vi "02 HEWH 24 Hour Test SM1.vi"(0 "Equipment":T1={"COM Port"="COM3", "MW100"="MW100", "AG34970"="A-34972A", "Chamber"="WT500"}, 2 "Semiphore":T2, 11 "Error In":errorcluster) -> (15 "Error Out":errorcluster)   [LabVIEW 2012]
uses:
  EquipReferences.ctl
  HEWH Tank Indicator.ctl
  PowerElements.ctl
  <vilib>/Platform/fileVersionInfo.llb/FileVersionInformation.ctl
  GEA2/HEWH_Mode.ctl
  ChannelSettings.ctl
  ValveBankPositions.ctl
  Intellifaucet/Intellfaucet Mode.ctl
  TestedFlowratesScenarios.ctl
  HEWH Error Enumeration.ctl
  <vilib>/Utility/file.llb/Write To Spreadsheet File (string).vi
  Global HEWH.vi
  <vilib>/Analysis/baseanly.llb/Mean (DBL).vi
  <vilib>/Analysis/NI_AALBase.lvlib
panel:
  in  "Tab Control":enum32{"Page 1", "Page 2"}(tab)
  in  "Time Reset":bool
  in  "Time Update":dbl format="%<%H:%M:%S>t"
  out "Tc Tree Check":dbl[](array[numeric]) format="%.4f"
  out "Serial Data In":string
  in  "IP Agilent":string="192.168.25.2"
  in  "IP MW100":string="192.168.25.4"
  in  "P2":i32=9
  in  "T5 2":i32=9
  in  "T2 2":i32=11
  in  "T1 2":i32=10
  in  "P5":i32=18
  in  "P1":i32=19
  out "Label Array":string[](array[string])
  out "Chanel List":string
  out "Computer Name":string
  in  "Stop Logging":bool
  in  "stop":bool
  out "StopSerial":bool
  out "FileVersionInfo Out":T3
  out "Calibration File Array":dbl[][](array[numeric])
  out "Flow Rate (GPM)":dbl
  out "Degrees F":dbl
  out "Voltage":dbl=240.0
  out "Number of Records":i32
  in  "Stop Test Seqence":bool
  out "Ver.":string
  out "Log Data":string[][](array[string])
  out "DrawCount":i32
  out "POWER":T4
  out "t*=0":dbl format="%<%H:%M:%S>t"
  out "Elapsed.Time (H:M:S)":dbl format="%<%H:%M:%S>t"
  out "STATUS":string
  in  "Help":bool
  out "Tank Display":T5 {"TC6" format="%.2g"; "TIN" format="%.2g"; "TOUT" format="%.2g"; "Mean" format="%.2f"; "Std Dev" format="%.2f"; "TC5" format="%.2g"; "TC4" format="%.2g"; "TC3" format="%.2g"; "TC2" format="%.2g"; "TC1" format="%.2g"}
  out "Current Draw Start Time":dbl format="%.2f"
  out "First Time":bool=TRUE
  out "Current State":string
  out "MW100":refnum<visa-resource-name>
  in  "Tab Control 2":enum32{"TEST STATUS", "DATA VIEW", "R134A P-H"}(tab)
  in  "Status Tabl":T6(tab)=enum."External Program Controls"
  in  "Read Config File":bool
  in  "RTDin to Downspout Offset":dbl
  in  "Power Off Time":dbl=82800.0 format="%<%H:%M>t"
  in  "End Log Duration":dbl=3600.0 format="%<%H:%M>t"
  in  "Config Filename":string="HEWH First Hour Rating.ini"
  in  "Num of PreDraws(0-3)":i32=1
  out "GEA2 HyperData":bool
  out "Data Array":string[][](array[string])
  in  "Expansion Tank?":bool
  out "Dispense Times":dbl[](array[numeric])=[0.0, 3600.0, 7200.0, 10800.0, 14400.0, 18000.0] format="%<%H:%M>t"
  out "Dispense Schedule":dbl[](array[numeric])=[10.72, 10.72, 10.72, 10.72, 10.72, 10.72] format="%.2f"
  out "Flow Rate Schedule":dbl[](array[numeric])=[3.0, 3.0, 3.0, 3.0, 3.0, 3.0] format="%.2f"
  out "Temperature Schedule":dbl[](array[numeric])=[58.0, 58.0, 58.0, 58.0, 58.0, 58.0] format="%.2f"
  in  "Cold Water Available?":bool=TRUE
  in  "T3":u32=500
  in  "T2":u32=150
  out "Local?":bool
  out "LAN IP Address":string="192.168.25.3"
  out "Init Complete":bool=TRUE
  in  "T1":u32=1000
  in  "T4":u32=30
  in  "T5":u32=50
  in  "Purge Guard Time(s)":dbl=360.0
  out "PowerON":bool=TRUE
  in  "Sample Per.(s)":dbl=5.0
  in  "Power Off Guard Time20s)":u32=20
  in  "Working File Directory":path=path "c:/work"
  out "Serial Port Available?":bool=TRUE
  out "COM Port":refnum<visa-resource-name>="COM3"
  in  "Save File Directory":path=path "c:/data"
  out "FileName":path
  out "Use Agilent?":bool
  out "GEA2 Set Mode":T7=enum."HighDemand"
  out "Set PointOut":u8=140
  in  "Calibration File":path=path "C:/work/CalibrationFile.csv"
  out "Calibration File?":bool
  out "Monitoring Temps Chart":T8(graph)
  out "Tcs 1-6":dbl[](array[numeric])
  in  "Purge Right Now":bool
  out "Downspount Flow":dbl(graph)
  out "Downspout Flow":dbl=3.8899999999999997
  out "Downspout Temp":dbl=76.8
  out "Temp Band(+/- F)":dbl=50.0
  out "Flow rate Adj":dbl=85.11482133995038
  out "Downspount Temp":dbl(graph)
  out "TempAdj":dbl
  out "Failed to Start Count":dbl
  in  "RTD Band":dbl=2.0
  in  "Skip Waiting for Cutout":bool
  in  "mean tank upper lim":dbl=140.0
  in  "meant tank lower lim":dbl=130.0
  out "Temp Range Err":bool=TRUE
  out "mean":dbl format="%0.2f"
  in  "Power Off Check Limit":dbl=20.0
  out "M*-1":dbl
  in  "Skip Waiting for Temp 3":bool
  out "Tcs 1-6, Ave. 3":dbl[](array[numeric])
  out "Temps Chart 2":T9(graph)
  in  "Temp Decline Hystersis":dbl=0.2
  out "T_Ave_Max":dbl
  out "T_Ave":dbl
  out "LastDraw":bool=TRUE
  out "T*Max":dbl
  out "Special Last Draw":bool
  out "Discard Last Draw":bool
  out "T*Ave":dbl
  out "T*min":dbl
  out "Volume(Gal.)":dbl
  in  "Flow Adj":dbl=3.0
  in  "Adj Time":dbl=3.0
  in  "K(0.1)":dbl=0.1
  out "TcDown":dbl
  out "Gal Target":dbl
  out "Drawing":bool=TRUE
  out "RTD Out":cluster{dbl, dbl}[](graph)
  out "Flowmeter":cluster{dbl, dbl}[](graph)
  in  "Skip Draw0":bool
  out "TcDown 0":dbl
  out "FlowMeter During Draw0":cluster{dbl, dbl}[](graph)
  out "RTD Out 0":cluster{dbl, dbl}[](graph)
  out "WattHours":dbl
  out "Total Gallons Drawn":dbl
  out "Error History":string[](array[string])
  out "Com History":string[](array[string])
  out "Test Data":dbl[][](array[numeric])
  out "Executaion Sequence":string[](array[string])
  out "Error Datalogging":errorcluster={"status"=TRUE, "code"=-1073807346, "source"="VISA Read in Gather Test Data.vi"}
  out "Serial Error Out":errorcluster
  out "Gallons Chart":dbl(graph)
  out "Temps":T8(graph) caption="Waveform Chart"
  out "Watt Chart":T10(graph)
  out "XY Graph":cluster{dbl[], dbl[]}[](graph)=[{array[3000 elements], array[3000 elements]}, {array[3000 elements], array[3000 elements]}, {array[3000 elements], array[3000 elements]}, {array[3000 elements], array[3000 elements]}, {array[3000 elements], array[3000 elements]}, {array[3000 elements], array[3000 elements]}, {array[3000 elements], array[3000 elements]}, {array[3000 elements], array[3000 elements]}, {array[3000 elements], array[3000 elements]}, {[-20.0, -19.0, -18.0, -17.0, -16.0, -15.0, -14.0, -13.0, -12.0, -11.0, -10.0, -9.0, -8.0, -7.0, -6.0, -5.0, -4.0, -3.0, -2.0, -1.0, 0.0, 1.0, 2.0, 3.0, 4.0, 5.0, 6.0, 7.0, 8.0, 9.0, 10.0, 11.0, 12.0, 13.0, 14.0, 15.0, 16.0, 17.0, 18.0, 19.0, 20.0, 21.0, 22.0, 23.0, 24.0, 25.0, 26.0, 27.0, 28.0, 29.0, 30.0, 31.0, 32.0, 33.0, 34.0, 35.0, 36.0, 37.0, 38.0, 39.0, 40.0, 41.0, 42.0, 43.0, 44.0, 45.0, 46.0, 47.0, 48.0, 49.0, 50.0, 51.0, 52.0, 53.0, 54.0, 55.0, 56.0, 57.0, 58.0, 59.0, 60.0, 61.0, 62.0, 63.0, 64.0, 65.0, 66.0, 67.0, 68.0, 69.0, 70.0, 71.0, 72.0, 73.0, 74.0, 75.0, 76.0, 77.0, 78.0, 79.0, 80.0, 81.0, 82.0, 83.0, 84.0, 85.0, 86.0, 87.0, 88.0, 89.0, 90.0, 91.0, 92.0, 93.0, 94.0, 95.0, 96.0, 97.0, 98.0, 99.0, 100.0, 101.0, 102.0, 103.0, 105.0, 106.0, 107.0, 108.0, 109.0, 110.0, 111.0, 112.0, 113.0, 114.0, 115.0, 116.0, 117.0, 118.0, 119.0, 120.0, 120.0, 119.0, 118.0, 117.0, 116.0, 115.0, 114.0, 113.0, 112.0, 111.0, 110.0, 109.0, 108.0, 107.0, 106.0, 105.0, 104.0, 103.0, 102.0, 101.0, 100.0, 99.0, 98.0, 97.0, 96.0, 95.0, 94.0, 93.0, 92.0, 91.0, 90.0, 89.0, 88.0, 87.0, 86.0, 85.0, 84.0, 83.0, 82.0, 81.0], [0.6289673515895778, 0.7335805994405737, 0.8522944773712947, 0.9865263135707176, 1.1377792235501054, 1.307642283538553, 1.497790359049673, 1.7099835899691802, 1.9460665393720367, 2.2079670150661914, 2.497694574185926, 2.8173387228323223, 3.1690668252624037, 3.5551217379777147, 3.9778191836295544, 4.439544882943048, 4.942751461266441, 5.489955147854285, 6.083732285515876, 6.726715668875549, 7.421590728326429, 8.171091577641509, 8.97799694218748, 9.845125983296143, 10.775334035813131, 11.771508272724029, 12.836563312210393, 13.97343677968726, 15.185084837974983, 16.47447769736936, 17.844595116102667, 19.298421901263723, 20.838943419302854, 22.469141123767677, 24.191988107816766, 26.010444687249684, 27.927454019633004, 29.94593776380572, 32.06879178324577, 34.29888189579838, 36.63903967202567, 39.09205828262364, 41.66068839552788, 44.34763412198737, 47.15554901030907, 50.08703208533592, 53.14462393080051, 56.330802811291676, 59.64798082967107, 63.09850011495871, 66.68462903565818, 70.40855843220261, 74.2723978613939, 78.27817184611749, 82.42781612136012, 86.72317386799375, 91.16599192444974, 95.75791696541866, 100.50049163628815, 105.3951506301971, 110.44321669390614, 115.64589654721868, 121.0042766986882, 126.51931913887094, 132.19185689016396, 138.02258938921167, 144.01207767566953, 150.16073935666577, 156.46884331294888, 162.93650410698515, 169.56367604908513, 176.35014686787835, 183.29553092825122, 190.39926192676901, 197.6605849865805, 205.07854806162732, 212.65199254633424, 220.3795429722877, 228.25959565629924, 236.29030614521017, 244.46957531341766, 252.79503371769874, 261.2640244979903, 269.8735838544667, 278.62041937927586, 287.50088568601166, 296.5109570183827, 305.64619643247437, 314.90172109495234, 324.2721631777093, 333.7516257565242, 343.33363303246585, 353.0110740850571, 362.776139234305, 372.62024791580313, 382.5339667649702, 392.5069163380596, 402.5276645496996, 412.5836045051322, 422.6608138540118, 432.74389199150977, 442.8157709281602, 452.85749412592986, 462.84795675360215, 472.76359917961935, 482.5780439241847, 492.26166554201416, 501.7810808394691, 511.09854992710956, 520.1712821280202, 528.9506547605449, 537.3813812499737, 545.4007215624794, 552.9379365977184, 559.914378684324, 566.2449292917087, 571.841952583963, 576.6234598723152, 580.5270985712426, 583.5301287032851, 585.6703799185226, 587.0558684337939, 587.8482742464494, 588.2187766112756, 588.141222950092, 587.7353480793577, 587.0045793932134, 585.8338297375634, 584.0814968868967, 581.5867381075718, 578.1703293860701, 573.6301970901309, 567.7314260012223, 560.1889447231491, 550.6375826543398, 538.5778811089474, 523.2676748961252, 503.4722250043322, 476.74287591689614, 436.1867525772887, 258.86825073563045, 212.9176680385524, 180.78139825830644, 155.55637925277966, 134.7894483242774, 117.24739581752505, 102.19594125822638, 89.15016413086498, 77.76637607585478, 67.78812451607219, 59.01641309414097, 51.29202031721926, 44.48438417488053, 38.48428826425407, 33.19886663207948, 28.548084395501796, 24.462191967965445, 20.879841214942935, 17.746663336307403, 15.014176320046165, 12.638931666532306, 10.581838530034458, 8.80762060419795, 7.284374267830785, 5.983204560636212, 4.877921811372575, 3.9447859917644017, 3.1622890688775986, 2.510967804825093, 1.973241282394523, 1.5332685483827069, 1.1768227163527458, 0.8911784857694051, 0.6650104734580355, 0.48830004815892614, 0.3522485547973939, 0.24919496943998803, 0.17253616510785447, 0.11664815838820218, 0.07680696216682602]}, {array[3001 elements], array[3000 elements]}, {array[3001 elements], array[3000 elements]}, {array[3001 elements], array[3000 elements]}, {array[3001 elements], array[3000 elements]}, {array[3001 elements], array[3000 elements]}, {array[3001 elements], array[3000 elements]}, {array[3001 elements], array[3000 elements]}, {array[3001 elements], array[3000 elements]}, {array[3001 elements], array[3000 elements]}, {array[3001 elements], array[3000 elements]}, {array[1497 elements], array[3000 elements]}, {array[367 elements], array[3000 elements]}, {[105.93255455967248, 112.42689092064614, 116.44273185991061, 119.39005203281901, 121.73245859730832, 123.68292155032175, 125.35769411781914, 126.82746233810603, 128.13852855165723, 129.32292887087297, 130.40377974295842, 131.39832632523272, 132.31978681701082, 133.1785229019096, 133.9828123095638, 134.73937583680953, 135.45374709219547, 136.1305382440235, 136.77363508519238, 137.38634288871017, 137.9714972706934, 138.53154969788162, 139.0686343109296, 139.58462076945574, 140.08115649531902, 140.55970077424976, 141.02155253358825, 141.46787315655828, 141.89970536328445, 142.3179889471939, 142.72357397660303, 143.11723193739945, 143.49966519146506, 143.87151504814895, 144.23336868651143, 144.58576511975667, 144.9292003570158, 145.2641318890312, 145.5909826015709, 145.91014420222888, 146.2219802316458, 146.52682871835324, 146.82500452681342, 147.11680144035168, 147.40249401419845, 147.68233923541382, 147.95657797198055, 148.22543634543274, 148.48912688834582, 148.74784962670168, 149.0017930486504, 149.2511349808856, 149.49604338303644, 149.73667706913432, 149.9731863640636, 150.20571370192226, 150.4343941723682, 150.65935744440003, 150.88072161924538, 151.09860542478617, 151.31311896234982, 151.52436712222354, 151.7324499617229, 151.93746291872876, 152.1394970978142, 152.33863955241046, 152.5349769894243, 152.72858456986066, 152.91954048386145, 153.10791792052248, 153.29378704341966, 153.47721515617653, 153.6582668568134, 153.8370041817833, 154.0134867405098, 154.18777184117317, 154.35991460841956, 154.52996809360934, 154.69798337816727, 154.86400967054675, 155.02809439727724, 155.19028328852437, 155.35062045855477, 155.50914848146851, 155.6659084625278, 155.82094010538827, 155.97428177551146, 156.12597056001817, 156.2760423242184, 156.4245317650394, 156.57147246155304, 156.71689692279, 156.86083663301557, 157.0033220946259, 157.14438286881423, 157.28404761414504, 157.42234412316537, 157.5592993571698, 157.69493947923266, 157.82928988560892, 157.9623752355998, 158.0942194799729, 158.2248458880204, 158.3542770733321, 158.4825350183574, 158.60964109782338, 158.7356161010718, 158.8604802533762, 158.98425323629277, 159.10695420709882, 159.22860181736635, 159.3492142307173, 159.46880913980348, 159.58740378255143, 159.70501495770998, 159.82165903973606, 159.93735199305377, 160.05210938571605], array[3000 elements]}, {[115.75648571045232, 122.96710483610089, 127.41110626220923, 130.66641496917595, 133.25017652577256, 135.39947386528175, 137.24353004774838, 138.86082490998805, 140.30271625314023, 141.60470877636496, 142.7924034889048, 143.88488704808177, 144.8967809236536, 145.83954100941116, 146.72231495787682, 147.55252673047508, 148.33628650994913, 149.07868521989295, 149.78401048432525, 150.45590830805375, 151.09750567473316, 151.71150605154946, 152.30025904127754, 152.8658272884191, 153.4100239317041, 153.9344590360081, 154.44055998118662, 154.9296063398964, 155.40274583643557, 155.861012710044, 156.305342289977, 156.736583295018, 157.1555082718746, 157.56282250128322, 157.95917163469338, 158.3451482731592, 158.72129765994984, 159.0881226267419, 159.44608790812475, 159.79562391905165, 160.13713007370498], array[3000 elements]}, {[126.64279203619105, 134.59551042073025, 139.48238407871023, 143.0559179261217, 145.88884682023712, 148.24327082708368, 150.26186226925034, 152.03117832205368, 153.60781194961234, 155.03086399858378, 156.32850606237244, 157.5217312777965, 158.626613306631, 159.65574014976434, 160.61915932787284], array[3000 elements]}, {[138.63130815699512, 147.35151057718, 152.69578330404357, 156.59768629350233, 159.68754798195272, 162.2533707275988], array[3000 elements]}, {[151.76064101738217, 161.27325812247335], array[3000 elements]}, {[28.52582270664602, 44.081568937286775, 114.09195514867488, 38.62915687641245, 28.534346175593843, 28.534346175593843, 112.64773025363029, 28.52582270664602], [85.14, 300.0, 103.58, 103.58, 103.58, 85.14, 85.14, 85.14]}] caption="R134a"
  out "P-T-H Data 2":dbl[][](array[numeric])=[[100.0, 300.0, 300.0, 300.0, 300.0, 100.0, 100.0], [100.0, 180.0, 159.82797496446995, 155.0455538281553, 90.0, 75.33598302783228, 79.98668044616512], [118.89390196078386, 128.58517593044672, 120.0, 66.38193229793575, 41.67786633925046, 41.67786633925046, 113.8316741703627]]
  out "Time":dbl
  # "24-HOUR RATING TEST"
  # "For Testing Purposes"
  # "Input HEWH Dispense Schedule. Standard Dispense time is 0-5 hours, 10.72 gallons/dispense @ 3 GPM and 58 Deg F."
  # "Wait for Cutout..."
  # "Input relays don't detect that UE or LE are on, and Power reading <\nCompressor LL (0.35 kW currently)"
  # "WAIT FOR TOP HEATER AND COMP OFF."
  # "T*max is max ave temp"
  # "Record output water temp after 15 secs, and at 5 sec intervals thereafter\nMonitor inlet water temp, must be 58 +/- 2 F\nTerminate draw when output temp = T*max -25F, record T*min"
  # "Terminate draw.  Record Tmin*, Tmax*, Tave* and M*"
  # "(For Last Draw, If after 30 sec, T< last tmin, stop and discard measurements, else continue)"
  # "1"
  # "2"
  # "3"
  # "4"
  # "5"
  # "6"
  # "7"
  # "P"
  # "T"
  # "H"
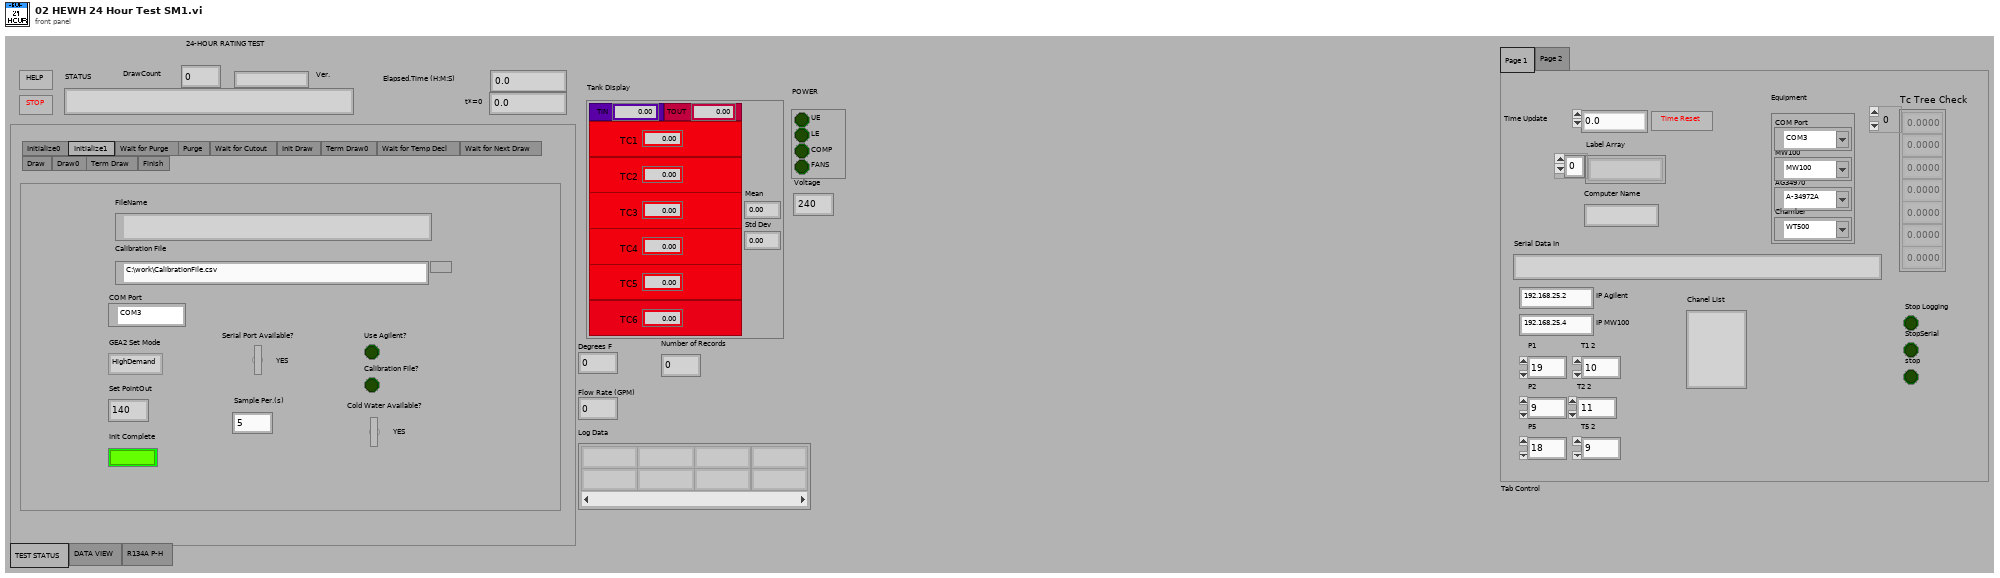
[diagram p1: front panel]
types:
  T1 = typedef "EquipReferences.ctl" = cluster{"COM Port":refnum<visa-resource-name>, "MW100":refnum<visa-resource-name>, "AG34970":refnum<visa-resource-name>, "Chamber":refnum<visa-resource-name>}
  T2 = typedef "Semaphore RefNum" = refnum<k1>
  T3 = typedef "FileVersionInformation.ctl" = cluster{"FileVersion":string, "ProductName":string, "InternalName":string, "CompanyName":string, "LegalCopyright":string, "FileDescription":string}
  T4 = typedef "PowerElements.ctl" = cluster{"UE":bool, "LE":bool, "COMP":bool, "FANS":bool}
  T5 = typedef "HEWH Tank Indicator.ctl" = cluster{"TC1-D":bool, "TC2-D":bool, "TC3-D":bool, "TC4-D":bool, "TC5-D":bool, "RTD_IN":bool, "RTDOUT":bool, "TC1":dbl, "TC2":dbl, "TC3":dbl, "TC4":dbl, "TC5":dbl, "TIN":dbl, "TOUT":dbl, "Std Dev":dbl, "Mean":dbl, "TC6-D":bool, "TC6":dbl}
  T6 = enum32{"Initialize0", "External Program Controls", "External Program Controls 2", "Program Controls", "Feedback", "Init Draw", "Feedback 2", "Feedback 3", "Feedback 4", "Draw", "Draw0", "Feedback 5", "Feedback 6"}
  T7 = typedef "HEWH_Mode.ctl" = enum16{"Hybrid", "StdElectric", "eHeat", "HighDemand", "Vacation"}
  T8 = cluster{"Tc Tree[0]":dbl, "Tc Tree[1]":dbl, "Tc Tree[2]":dbl, "Tc Tree[3]":dbl, "Tc Tree[4]":dbl, "Tc Tree[5]":dbl}[]
  T9 = cluster{"[0]":dbl, "[1]":dbl, "[2]":dbl, "[3]":dbl, "[4]":dbl, "[5]":dbl, "[6]":dbl}[]
  T10 = cluster{"[0]":dbl, "[1]":dbl, "[2]":dbl, "[3]":dbl, "[4]":dbl, "[5]":dbl}[]
  T11 = typedef "Intellfaucet Mode.ctl" = enum16{"Adjust Temp", "Adjust Flow", "Start Flow", "Stop Flow"}
  T12 = typedef "ValveBankPositions.ctl" = enum16{"Heating", "Purge", "Resting", "Draw"}
  T13 = typedef "TestedFlowratesScenarios.ctl" = enum16{"DRK500,Station1", "DRK375,Lab", "SRK500,Station1,5GPM FR", "DRK375,STATION3,1/2\"HOSE", "DRK500,Station1,downspout", "DRK375,Station3,thruEcocute", "DRK375,Station3,purge", "Build2,2B,Purge", "Global, Purge", "Global, Tank"}
  T14 = typedef "HEWH Error Enumeration.ctl" = enum16{"No Error", "GEA2 Send ACK Mismatch", "GEA2 STX", "GEA2 ETX", "GEA2 CRC Mismatch", "GEA2 ReadACK", "RTD In Range Error", "Fail Mean Tank Temp", "No Flow Config Data Found", "Failed Flow During Purge", "Temp During Purge", "Confirm IF Stop Fail", "Init Draw: TC_1 Out of Range", "Flow = 0 During Draw after 20s"}
  T15 = enum16{"Computation Start", "Computation stop", "Reset Computation", "Clear Computation"}
  T16 = cluster{" Draw Test Condition":enum16{"DRK500,Station1", "DRK375,Lab", "SRK500,Station1,5GPM FR", "DRK500,Station1,downspout"}, "Serial Port Available?":bool, "Cold Water Available?":bool, "TempErLimit":dbl, "Temp Decline Hystersis":dbl, "Target IP Address":string}
  T17 = cluster{"Degree Setting":dbl, "Flow rate setting":dbl, "Tc1 LL":dbl, "Tc1 UL":dbl}
  T18 = cluster{"No Serial  Sample Period(s)":dbl, "T5":u32, "T4":u32, "T1":u32, "T2":u32, "T3":u32}
  T19 = typedef "Cluster Purge Settings.ctl" = cluster{"Temp SettleTimeLimit(S)":dbl, "Steady State Persist Time(mS)":u32, "Purge Min Time":i32, "Flow SettleTimeLimit(S)":dbl, "Flow Adjust Time (3s)":dbl, "Flow Band (+/-GPM)":dbl, "Proportional Control Adjust Rate":dbl}
  T20 = cluster{"PurgreTempLimit":dbl, "Purge Condition TC":enum16{"TC1", "TC2", "TC3", "TC4", "TC5", "TC6"}, "Purgre0TempLim":dbl, "Purge Guard Time(s)":dbl}
  T21 = enum16{"Computation Start", "Computation stop", "Reset Computation", "Clear Computation"}[]
  T22 = cluster{"Tc Tree[0]":dbl, "Tc Tree[1]":dbl, "Tc Tree[2]":dbl, "Tc Tree[3]":dbl, "Tc Tree[4]":dbl, "Tc Tree[5]":dbl}
  T23 = cluster{"[0]":dbl, "[1]":dbl, "[2]":dbl, "[3]":dbl, "[4]":dbl, "[5]":dbl, "[6]":dbl}
  T24 = typedef "PowerData.ctl" = cluster{"Voltage":dbl, "Current":dbl, "Power":dbl, "WattHours":dbl}
  T25 = typedef "ChannelSettings.ctl" = u32
  T26 = cluster{"[0]":dbl, "[1]":dbl, "[2]":dbl, "[3]":dbl, "[4]":dbl, "[5]":dbl}
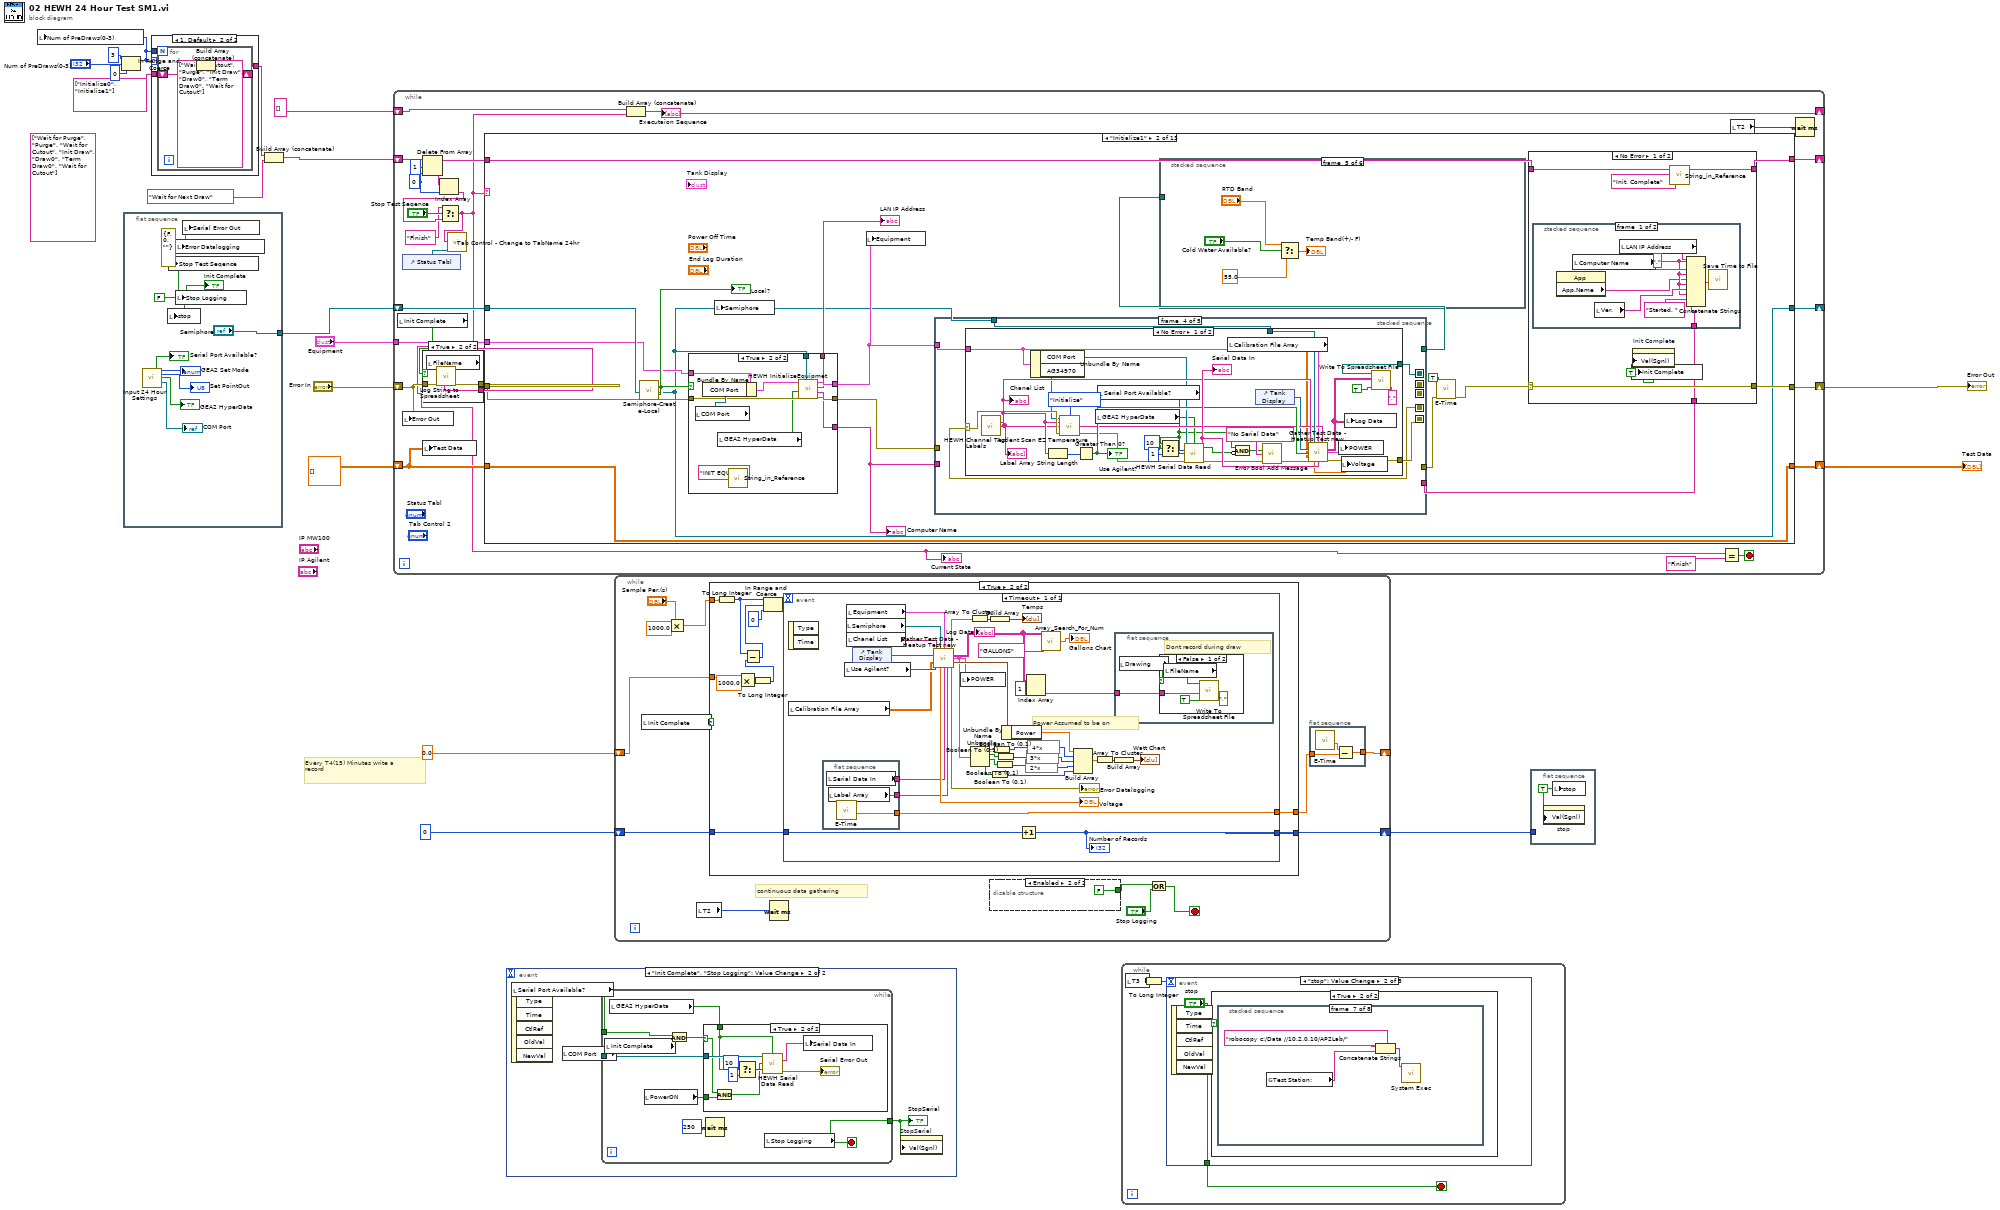
[diagram p0: block diagram]
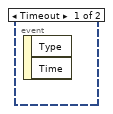
[diagram p2: hidden frame]
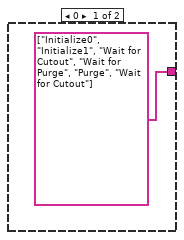
[diagram p4: hidden frame]
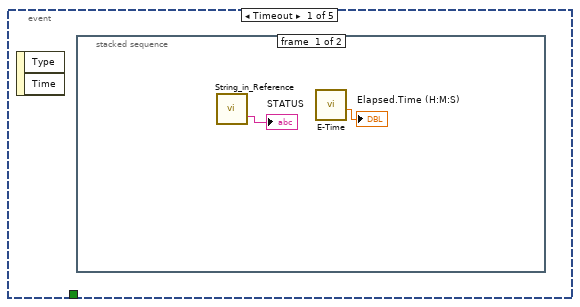
[diagram p5: hidden frame]
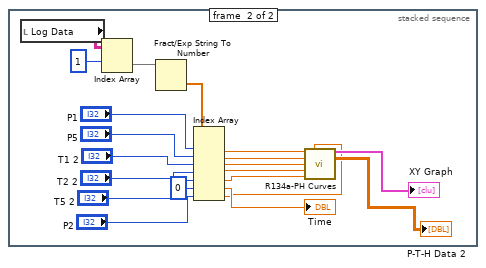
[diagram p6: hidden frame]
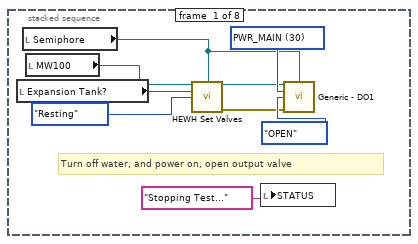
[diagram p8: hidden frame]
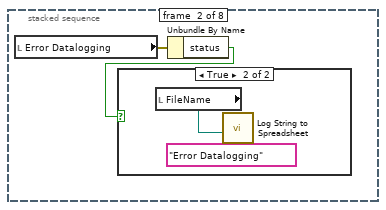
[diagram p9: hidden frame]
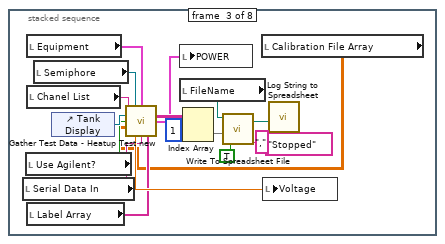
[diagram p11: hidden frame]
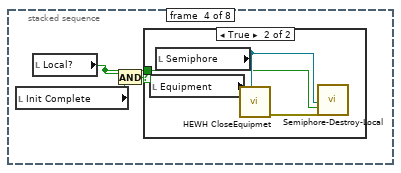
[diagram p12: hidden frame]
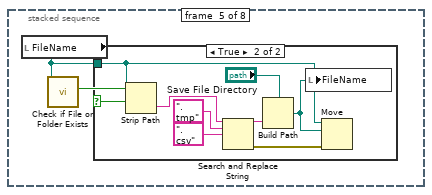
[diagram p14: hidden frame]
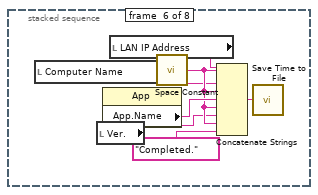
[diagram p16: hidden frame]
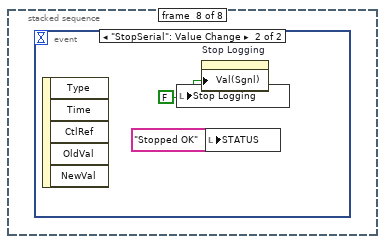
[diagram p17: hidden frame]
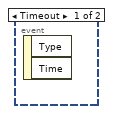
[diagram p18: hidden frame]
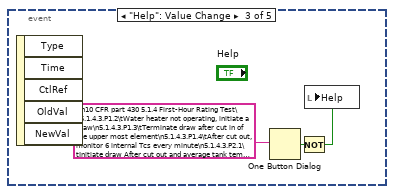
[diagram p19: hidden frame]
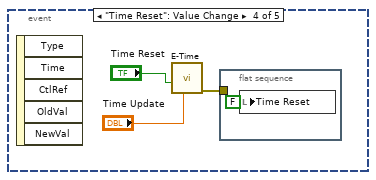
[diagram p20: hidden frame]
diagram:
  (unwired) string[] ["Wait for Purge", "Purge", "Wait for Cutout", "Init Draw", "Draw0", "Term Draw0", "Wait for Cutout"]
  # "Every T4(15) Minutes write a \nrecord"
  n1 = In Range and Coerce(upper limit=3, x="Num of PreDraws(0-3)", lower limit=0) -> (coerced(x)=w4:i32)  [unwired: 1 out]
  n2 = local write "Num of PreDraws(0-3)"(w4) -> ()
  n3 = flat-sequence {
    tunnel: ["Semiphore"] -> w16
    frame #0 {
      w24 = errorcluster {"status"=FALSE, "code"=0, "source"=""} ("errordatalogging")
      w25 = FALSE ("First Time 2")
      n4 = call "Input 24 Hour Settings.vi"() -> ("Serial Port Available?"=→"Serial Port Available?":bool, "GEA2 Set Mode Out"=→"GEA2 Set Mode":T7, "Set PointOut"=→"Set PointOut":u8, "GEA2 HyperData Out"=→"GEA2 HyperData":bool, "COM Port Out"=→"COM Port":refnum<visa-resource-name>)  [unwired: 10 in, 1 out]
      n5 = local write "stop"(w25) -> ()
      n6 = local write "Stop Test Seqence"(w25) -> ()
      n7 = local write "Error Datalogging"(w24) -> ()
      n8 = local write "Stop Logging"(w25) -> ()
      n9 = local write "Serial Error Out"(w24) -> ()
      "Init Complete" <- w25
    }
  }
  n10 = case shown="1, Default" w4 {
    tunnel: [string[] ["Initialize0", "Initialize1", "Wait for Cutout", "Wait for Purge", "Purge", "Wait for Cutout"] w30] -> w10
    tunnel: string[] ["Initialize0", "Initialize1"] -> [_ w29]
    tunnel: w4 -> [_ w28]
    frame 0 {
    }
    frame 1, Default {
      n11 = for {
        N: w28 -> [_]
        shift-right: [w31] -> w30
        shift-left: w29 -> [w33]
        n12 = Build Array (concatenate)(w33, string[] ["Wait for Cutout", "Purge", "Init Draw", "Draw0", "Term Draw0", "Wait for Cutout"]) -> (w31:string[])
      }
    }
  }
  n13 = Build Array (concatenate)(w10, "Wait for Next Draw") -> (w5:string[])
  n14 = while {
    shift-right: [w55] -> _
    shift-left: w5 -> [w58]
    shift-right: [w53] -> w17
    shift-left: "Error In" -> [w41]
    tunnel: "Equipment" -> [w49]
    shift-right: [w48] -> w14
    shift-left: dbl[][] [] -> [w47]
    shift-right: [w46] -> _
    shift-left: w16 -> [w50]
    shift-right: [w42] -> _
    shift-left: string[] [] -> [w43]
    stop <- w52 stop-if-true
    w45 = 0 ("index")
    n15 = local read "Init Complete"() -> (w39:bool)
    n16 = local write "Error Out"(w41) -> ()
    n17 = control-ref of="Status Tabl"() -> (w38:refnum<vi>)
    n18 = Delete From Array(array=w58, length=1, index=w45) -> (deleted portion=w56:string[], array with subset deleted=w54:string[])
    n19 = local write "Test Data"(w47) -> ()
    n20 = Index Array(array=w56, index=w45) -> (element=w36:string)
    n21 = Select(t="Finish" ("y"), s="Stop Test Seqence", f=w36) -> (s? t:f=w35:string)
    "Current State" <- w35
    n22 = case shown="True" w39 {
      tunnel: w41 -> [w59 w62]
      tunnel: [w59 w61] -> w40
      tunnel: w35 -> [_ w60]
      frame False {
      }
      frame True {
        n23 = local read "FileName"() -> (w63:path)
        n24 = call "Log String to Spreadsheet.vi"("String"=w60, "error in (no error)"=w62, "FileName"=w63) -> ("error out"=w61:errorcluster)  [unwired: 8 in]
      }
    }
    n25 = call "Tab Control - Change to TabName 24hr.vi"("Label.Text"=w35, "Status Tabl 3"=w38) -> ()  [unwired: 9 in]
    n26 = case shown="\"Initialize1\"" w35 {
      selector: w35 -> [_ _ _ _ _ _ _ _ _ _ _ _ w1182]
      tunnel: [w72 w115 w310 w387 w444 w564 w635 w700 w714 w892 w1033 w1148 w1197] -> w55
      tunnel: w54 -> [w72 w116 w311 w385 w442 w562 w636 w701 _ w893 w1033 w1149 w1196]
      tunnel: [w67 w113 w309 w386 w443 w563 w634 w699 w716 w890 w1034 w1147 w1183] -> w53
      tunnel: w40 -> [_ w114 w306 w378 w436 w547 w612 w697 w712 w894 w1031 w1119 w1184]
      tunnel: w50 -> [w73 w112 w313 w367 w440 w555 w617 w688 w713 w901 w1035 w1123 w1181]
      tunnel: w49 -> [_ w111 w312 w388 _ w554 _ _ _ w896 w1029 _ w1195]
      tunnel: [w74 w110 w314 w384 w441 w561 w637 w698 w715 w898 w1032 w1146 w1194] -> w48
      tunnel: w47 -> [w74 w110 w314 w384 w441 w561 w637 w698 w715 w898 w1032 w1145 w1194]
      tunnel: [w73 w103 w313 w367 w440 w555 w617 w688 w713 w897 w1030 w1123 w1181] -> w46
      frame "Initialize0" {
        w71 = FALSE ("Tool Bar:Show Abort Button")
        n27 = property class="VI"("TB.ShowAbortBut"=w71) -> ()  [unwired: 2 in, 2 out]
        n28 = property class="VI"("TB.ShowFreeRunBut"=w71) -> ()  [unwired: 2 in, 2 out]
        n29 = Current VI's Path() -> (path=w81:path)
        n30 = call "This VIs Path.vi"("path"=w81) -> ("current path"=w76:path, "File Version Info"=→"Ver.":string, "FileVersionInfo Out"=→"FileVersionInfo Out":T3, "error out"=w80:errorcluster)  [unwired: 10 in, 1 out]
        n31 = Build Path(base path=w76, name or relative path="Config Filename") -> (appended path=w79:path)
        n32 = case shown="True" "Read Config File" {
          tunnel: w79 -> [_ w90]
          tunnel: w80 -> [w82 w86]
          tunnel: [w82 w85] -> w68
          frame False {
          }
          frame True {
            n33 = call "Config File 24 Hour Test.vi"("Config File Path"=w90, "Error In"=w86) -> ("Test Condition Settings Cluster"=w89:T16, "DOE Test Spec Settings Cluster"=w88:T17, "Timing Cluster"=w87:T18, "Purge Settings Cluster"=w83:T19, "Purge Condition Settings Cluster"=w84:T20, "Error Out"=w85:errorcluster)  [unwired: 8 in]
            n34 = stacked-sequence {
              tunnel: w89 -> [w91 _ _ _ _ _]
              tunnel: w88 -> [_ w93 _ _ _ _]
              tunnel: w87 -> [_ _ w94 _ _ _]
              tunnel: [_ w92 _ _ _ _] -> _
              tunnel: w85 -> [_ _ _ _ _ w97]
              tunnel: w84 -> [_ _ _ _ w96 _]
              tunnel: w83 -> [_ _ _ w95 _ _]
              frame #0 {
                n35 = Unbundle(w91) -> ()  [unwired: 6 out]
              }
              frame #1 {
                n36 = Unbundle(w93) -> ("Flow rate setting"=w92:dbl)  [unwired: 3 out]
              }
              frame #2 {
                n37 = Unbundle(w94) -> ()  [unwired: 6 out]
              }
              frame #3 {
                n38 = Unbundle By Name(w95) -> ()  [unwired: 2 out]
              }
              frame #4 {
                n39 = Unbundle(w96) -> ()  [unwired: 4 out]
              }
              frame #5 {
                n40 = case shown="Error" w97 {
                  frame No Error {
                  }
                  frame Error {
                    n41 = call <vilib>:"Simple Error Handler.vi"("error in (no error)"=errorcluster {"status"=TRUE, "code"=-7600, "source"="Config File Error"}) -> ()  [unwired: 4 in, 5 out]
                    n42 = Stop(stop? (T)=TRUE) -> ()
                  }
                }
              }
            }
          }
        }
        n43 = call "String_in_Reference.vi"("String"="Initializing") -> ()  [unwired: 18 in, 1 out]
        n44 = call "Calibration File Check.vi"("error in (no error)"=w68, "Calibration Path"="Calibration File") -> ("error out"=w67:errorcluster, "Calibration File Array"=→"Calibration File Array":dbl[][], "Complete File?"=→"Calibration File?":bool)  [unwired: 6 in, 1 out]
      }
      frame "Initialize1" {
        n45 = call "Semiphore-Create-Local.vi"("Semiphore"=w112, "error in (no error)"=w114) -> ("semaphore"=w103:T2, "Local?"=w117:bool, "error out"=w118:errorcluster)  [unwired: 15 in]
        "Local?" <- w117
        n46 = case shown="True" w117 {
          tunnel: w118 -> [w289 w292]
          tunnel: [w288 w299] -> w106
          tunnel: [w289 w300] -> w105
          tunnel: w111 -> [w288 w297]
          tunnel: w103 -> [_ w293]
          tunnel: [w287 w296] -> w109
          tunnel: [w286 w295] -> w104
          frame False {
            n47 = call "IP and Computer Name.vi"() -> ("IP Address"=w287:string, "Computer Name"=w286:string)  [unwired: 10 in]
          }
          frame True {
            n48 = local read "COM Port"() -> (w294:refnum<visa-resource-name>)
            n49 = Bundle By Name(cluster=w297, "COM Port"=w294) -> (w291:T1)
            n50 = local read "GEA2 HyperData"() -> (w290:bool)
            n51 = call "String_in_Reference.vi"("String"="INIT EQUIP") -> ()  [unwired: 18 in, 1 out]
            n52 = call "HEWH InitializeEquipmet.vi"("Semiphore"=w293, "Error In"=w292, "GEA2?"=w290, "Equipment"=w291) -> ("Error Out"=w300:errorcluster, "Computer Name"=w295:string, "LAN IP Address"=w296:string, "Equipment Out"=w299:T1)  [unwired: 4 in]
          }
        }
        "LAN IP Address" <- w109
        "Computer Name" <- w104
        n53 = local write "Semiphore"(w103) -> ()
        n54 = local write "Equipment"(w106) -> ()
        n55 = stacked-sequence {
          seq-local: [_ _ w174 _ _] -> [_ _ _ w187 _]
          seq-local: [_ w135 _ _ _] -> [_ _ w178 _ _]
          seq-local: [_ _ _ w189 _] -> [_ _ _ _ w228]
          seq-local: [_ w134 _ _ _] -> [_ _ _ w188 _]
          seq-local: [w123 _ _ _ _] -> [_ w141 _ _ _]
          tunnel: [_ _ _ _ w224] -> w101
          tunnel: w104 -> [_ w144 _ _ _]
          tunnel: w105 -> [w122 _ _ _ _]
          tunnel: w106 -> [w121 w137 w186 w191 w227]
          tunnel: w103 -> [_ _ w173 w190 w225]
          tunnel: [_ w134 _ _ _] -> w102
          tunnel: [_ w148 _ _ _] -> w100
          frame #0 {
            # "Read globals.  Used in file init routine."
            n56 = Unbundle By Name(w121) -> ("COM Port"=w120:refnum<visa-resource-name>)
            n57 = local read "GEA2 HyperData"() -> (w119:bool)
            n58 = case shown="False" w119 {
              tunnel: [w124 w129] -> w123
              tunnel: w122 -> [w124 w128]
              tunnel: w120 -> [_ w127]
              frame False {
              }
              frame True {
                n59 = local read "GEA2 Set Mode"() -> (w125:T7)
                n60 = local read "Set PointOut"() -> (w126:u8)
                n61 = call "HEWH GEA2 Set Tank Mode and Temp.vi"("ComPort"=w127, "Mode"=w125, "Set Point"=w126, "Error In"=w128) -> ("Error Out"=w129:errorcluster)  [unwired: 9 in, 2 out]
              }
            }
          }
          frame #1 {
            # "File init uses globals."
            # "Initialize Data file ."
            n62 = local read "FileVersionInfo Out"() -> (w146:T3)
            n63 = local read "GEA2 Set Mode"() -> (w131:T7)
            n64 = local read "Set PointOut"() -> (w138:u8)
            n65 = Unbundle By Name(w137) -> ("COM Port"=w136:refnum<visa-resource-name>)
            n66 = Unbundle By Name(w146) -> ("FileVersion"=w145:string)  [unwired: 1 out]
            n67 = case shown="\"Hybrid\", Default" w131 {
              tunnel: ["SE" ("Mode:") "EH" ("Mode:") "HD" ("Mode:") "HY" ("Mode:")] -> w132
              frame "StdElectric" {
              }
              frame "eHeat" {
              }
              frame "HighDemand" {
              }
              frame "Hybrid", Default {
              }
            }
            n68 = call "HEWH Data File Info String.vi"("Set PointOut"=w138, "GEA2 Set Mode"=w131) -> ("Info string"=w139:string)  [unwired: 9 in]
            n69 = local read "GEA2 HyperData"() -> (w130:bool)
            n70 = call "Data_File_Init.vi"("Data File Directory"="Working File Directory", "Test_Name In:"="24DOE", "Version In:"=w145, "Computer Name In:"=w144, "error in (no error)"=w141, "File Extension:"="tmp", "Ambient Temp / RH:"=w139, "Mode:"=w132) -> ("FileName"=w134:path, "Data Array"=w147:string[][], "error out"=w140:errorcluster)  [unwired: 5 in]
            "FileName" <- w134
            "Data Array" <- w147
            n71 = case shown="True" w130 {
              tunnel: w140 -> [w151 w157]
              tunnel: w136 -> [_ w156]
              tunnel: [w151 w155] -> w135
              tunnel: w134 -> [_ w152]
              frame False {
              }
              frame True {
                n72 = call "GEA2_RQST_SOFTWARE_VER.vi"("ComPort"=w156, "Error In"=w157) -> ("Software Version"=w153:string, "Error Out"=w154:errorcluster)  [unwired: 10 in, 2 out]
                n73 = call "Log String to Spreadsheet.vi"("String"=w153, "error in (no error)"=w154, "FileName"=w152) -> ("error out"=w155:errorcluster)  [unwired: 8 in]
              }
            }
            n74 = Array To Spreadsheet String(delimiter (Tab)=",", array=w147, 3:"%s" ("format string")) -> (spreadsheet string=w148:string)
          }
          frame #2 {
            # "Solenoid Out+com port turns the com port off that controls the \ngallon calc. Turns off Gal Calc, initially."
            # "Set Valves."
            n75 = local read "DrawCount"() -> (w166:i32)
            n76 = call "Dispense Schedule.vi"() -> ("Dispense Times"=→"Dispense Times":dbl[], "Dispense Schedule"=→"Dispense Schedule":dbl[], "Flow Rate Schedule"=w164:dbl[], "Temperature Schedule"=w165:dbl[])  [unwired: 6 in]
            "Temperature Schedule" <- w165
            "Flow Rate Schedule" <- w164
            n77 = Unbundle(w186) -> ("MW100"=w184:refnum<visa-resource-name>)  [unwired: 3 out]
            "MW100" <- w184
            n78 = Index Array(array=w165, index=w166) -> (element=→"Degrees F":dbl)
            n79 = Index Array(array=w164, index=w166) -> (element=→"Flow Rate (GPM)":dbl)
            n80 = call "HEWH Set Valves.vi"("VISA session"=w184, "Semiphore"=w173, "Expansion Tank?"="Expansion Tank?", "Valve Bank Setting"=ValveBankPositions."Heating", "Error In"=w178) -> ("dup VISA session"=w183:refnum<visa-resource-name>, "Error Out"=w182:errorcluster)  [unwired: 9 in]
            n81 = local read "Flow Rate (GPM)"() -> (w168:dbl)
            n82 = call "HEWH Totalize Flow Control.vi"("VISA session"=w183, "Semiphore"=w173, "Totalize Flow"=FALSE, "error in (no error)"=w182) -> ("dup VISA session"=w176:refnum<visa-resource-name>, "error out"=w179:errorcluster)  [unwired: 10 in]
            n83 = call "Intellifaucet_Driver.vi"("VISA session"=w176, "Mode"=Intellfaucet_Mode."Adjust Flow", "Semiphore"=w173, "Percent Flow"=w168, "Error In"=w179) -> ("VISA session out"=w171:refnum<visa-resource-name>, "Error Out"=w177:errorcluster)  [unwired: 9 in]
            n84 = local read "Degrees F"() -> (w167:dbl)
            n85 = call "Intellifaucet_Driver.vi"("VISA session"=w171, "Mode"=Intellfaucet_Mode."Adjust Temp", "Semiphore"=w173, "Temperature(F)"=w167, "Error In"=w177) -> ("Error Out"=w174:errorcluster)  [unwired: 9 in, 1 out]
          }
          frame #3 {
            n86 = case shown="No Error" w187 {
              selector: w187 -> [w222 w223]
              tunnel: w191 -> [w212 _]
              tunnel: w190 -> [w216 _]
              tunnel: [w209 w223] -> w189
              tunnel: w188 -> [w205 _]
              frame No Error {
                n87 = call "HEWH Channel Test Labels.vi"() -> ("Chanel List"=w217:string, "Label List"=w215:string[])  [unwired: 13 in, 1 out]
                "Chanel List" <- w217
                "Label Array" <- w215
                n88 = Unbundle By Name(w212) -> ("COM Port"=w211:refnum<visa-resource-name>, "AG34970"=w210:refnum<visa-resource-name>)
                n89 = String Length(string=w217) -> (length=w220:i32)
                n90 = call "Agilent Scan EZ Temperature.vi"("VISA Resource Name"=w210, "Control"=enum16{"Initialize", "Read", "Experiment"}."Initialize", "Channel Input"=w217, "error in (no error)"=w222) -> ("error out"=w213:errorcluster)  [unwired: 8 in, 3 out]
                n91 = Greater Than 0?(x=w220) -> (x > 0?=w218:bool)
                "Use Agilent?" <- w218
                n92 = local read "GEA2 HyperData"() -> (w196:bool)
                n93 = local read "Serial Port Available?"() -> (w193:bool)
                n94 = Select(t=10, s=w193, f=1) -> (s? t:f=w200:i32)
                n95 = call "HEWH Serial Data Read.vi"("Serial Port Ref"=w211, "GEA2 HyperData"=w196, "Retries"=w200, "Serial Port Available?"=w193, "error in (no error)"=w213) -> ("Serial Read OK"=w194:bool, "Read String"=w219:string, "error out"=w199:errorcluster)  [unwired: 7 in, 1 out]
                "Serial Data In" <- w219
                n96 = local read "Calibration File Array"() -> (w192:dbl[][])
                n97 = Compound Arithmetic op=AND(w193, invert w194) -> (w195:bool)
                n98 = control-ref of="Tank Display"() -> (w204:refnum<vi>)
                n99 = call "Error Bool Add Message.vi"("Error?"=w195, "Message"="No Serial Data", "Error In"=w199) -> ("Error Out"=w198:errorcluster)  [unwired: 12 in]
                n100 = call "Gather Test Data - Heatup Test new.vi"("Agilent Scan List"=w217, "Semiphore"=w216, "Equipment"=w212, "Tank Display Ref"=w204, "Agilent?"=w218, "Calibration Coefficients"=w192, "error in (no error)"=w198, "Serial Data In"=w219, "Agilent Label Array"=w215) -> ("Output Data"=w206:string[][], "POWER"=w214:T4, "Voltage"=w203:dbl, "error out"=w209:errorcluster)  [unwired: 1 in, 2 out]
                n101 = local write "POWER"(w214) -> ()
                n102 = local write "Voltage"(w203) -> ()
                n103 = local write "Log Data"(w206) -> ()
                n104 = call-poly <vilib>:"Write To Spreadsheet File.vi"("delimiter (\\t)"="," ("delimiter (\\t)"), "append to file? (new file:F)"=TRUE, "2D data"=w206, "file path (dialog if empty)"=w205) -> ()  [unwired: 4 in, 1 out]
              }
              frame Error {
              }
            }
          }
          frame #4 {
            w229 = T21 [enum."Computation Start", enum."Reset Computation"] items=["Computation Start", "Computation stop", "Reset Computation", "Clear Computation"]
            # "Reset and restart computation of gallons."
            n105 = Unbundle By Name(w227) -> ("MW100"=w226:refnum<visa-resource-name>)
            n106 = for {
              tunnel: w229 -> [w232] mode=indexing
              shift-right: [w233] -> w224
              shift-left: w228 -> [w234]
              tunnel: w225 -> [w231]
              tunnel: w226 -> [w230]
              n107 = call "YKMW100 Computation Control.vi"("VISA session"=w230, "Semiphore"=w231, "Mode"=w232, "error in (no error)"=w234) -> ("error out"=w233:errorcluster)  [unwired: 10 in, 1 out]
            }
          }
        }
        n108 = stacked-sequence {
          tunnel: w102 -> [_ _ _ _ _ w256]
          frame #0 {
            # "Clear Charts."
            n109 = property on="Temps Chart 2" class="WFChart (strict)"("History Data"=T9 []) -> ()  [unwired: 2 in, 2 out]
            n110 = property on="Watt Chart" class="WFChart (strict)"("History Data"=T10 []) -> ()  [unwired: 2 in, 2 out]
            n111 = property on="Monitoring Temps Chart" class="WFChart (strict)"("History Data"=T8 []) -> ()  [unwired: 2 in, 2 out]
            n112 = property on="Temps" class="WFChart (strict)"("History Data"=T8 []) -> ()  [unwired: 2 in, 2 out]
            n113 = property on="Gallons Chart" class="WFChart (strict)"("History Data"=dbl[] []) -> ()  [unwired: 2 in, 2 out]
            "DrawCount" <- 0
          }
          frame #1 {
            # "Flow Loop Time"
            # "30 Second Delay between Samples thru test"
            # "UI Refresh Rate"
            # "Loop Delays, prevent overwork Machine"
            # "Sample Period for Decision Data"
            "t*=0" <- 0.0 ("t*=0")
          }
          frame #2 {
            w242 = dbl[] [] ("History Data")
            n114 = local write "Power Off Guard Time20s)"(u32 20 ("Power Off Guard Time")) -> ()
            n115 = local write "Failed to Start Count"(0.0 ("Failed to Start Count")) -> ()
            n116 = property on="Downspount Temp" class="WFChart (strict)"("History Data"=w242) -> ()  [unwired: 2 in, 2 out]
            n117 = property on="Downspount Flow" class="WFChart (strict)"("History Data"=w242) -> ()  [unwired: 2 in, 2 out]
          }
          frame #3 {
            w246 = TRUE ("First Time")
            w245 = FALSE ("BottomHeater")
            n118 = local write "Temp Range Err"(w245) -> ()
            n119 = local write "Drawing"(w245) -> ()
            n120 = local write "Skip Waiting for Cutout"(w245) -> ()
            n121 = local write "Purge Right Now"(w245) -> ()
            n122 = local write "Skip Draw0"(w245) -> ()
            n123 = local write "Time Reset"(w245) -> ()
            n124 = local write "LastDraw"(w245) -> ()
            n125 = local write "Help"(w245) -> ()
            n126 = local write "POWER"(T4 {"UE"=FALSE, "LE"=FALSE, "COMP"=FALSE, "FANS"=FALSE} ("POWER 2")) -> ()
            "First Time" <- w246
            "Special Last Draw" <- w245
            "Discard Last Draw" <- w245
            "PowerON" <- w246
          }
          frame #4 {
            n127 = Select(t="RTD Band", s="Cold Water Available?", f=55.0) -> (s? t:f=→"Temp Band(+/- F)":dbl)
          }
          frame #5 {
            n128 = local read "Dispense Schedule"() -> (w253:dbl[])
            n129 = local read "Dispense Times"() -> (w252:dbl[])
            n130 = Number To Fractional String(number=w252) -> (F-format string=w262:string[])  [unwired: 3 in]
            n131 = Build Array (concatenate)("Dispense Times" ("string"), w262) -> (w264:string[])
            n132 = call-poly <vilib>:"Write To Spreadsheet File.vi"("delimiter (\\t)"="," ("delimiter (\\t)"), "append to file? (new file:F)"=TRUE, "1D data"=w264, "file path (dialog if empty)"=w256) -> ("new file path (Not A Path if cancelled)"=w255:path)  [unwired: 4 in]
            n133 = Number To Fractional String(number=w253) -> (F-format string=w261:string[])  [unwired: 3 in]
            n134 = Build Array (concatenate)("Dispense Schedule" ("string"), w261) -> (w260:string[])
            n135 = call-poly <vilib>:"Write To Spreadsheet File.vi"("delimiter (\\t)"="," ("delimiter (\\t)"), "append to file? (new file:F)"=TRUE, "1D data"=w260, "file path (dialog if empty)"=w255) -> ()  [unwired: 4 in, 1 out]
            "T*Max" <- 0.0 ("T*Max")
            "T*min" <- 1000.0 ("T*min")
          }
        }
        n136 = call "E-Time.vi"("error in (no error)"=w101, "Reset"=TRUE) -> ("error out"=w107:errorcluster)  [unwired: 7 in, 2 out]
        n137 = case shown="No Error" w107 {
          selector: w107 -> [w272 w285]
          tunnel: [w271 string[] ["Finish"] ("States")] -> w115
          tunnel: [w272 w285] -> w113
          tunnel: w116 -> [w271 _]
          tunnel: w100 -> [w269 _]
          frame No Error {
            w268 = TRUE ("Init Complete")
            n138 = stacked-sequence {
              tunnel: w269 -> [w273 _]
              frame #0 {
                w277 = ","
                n139 = property class="App"() -> ("App.Name"=w276:string)  [unwired: 2 in, 2 out]
                n140 = local read "Computer Name"() -> (w280:string)
                n141 = local read "Ver."() -> (w279:string)
                n142 = local read "LAN IP Address"() -> (w275:string)
                n143 = Concatenate Strings(w275, w277, w280, w277, w276, w277, w279, w277, "Started. " ("string"), w273) -> (w274:string)
                n144 = call "Save Time to File.vi"("String"=w274) -> ()  [unwired: 13 in, 2 out]
              }
              frame #1 {
                n145 = global read "Global HEWH.vi" "Test Station:"() -> (w282:string)
                n146 = Concatenate Strings("robocopy c:/Data //10.2.0.10/AP2Lab/" ("command line"), w282) -> (w283:string)
                n147 = call <vilib>:"System Exec.vi"("command line"=w283) -> ()  [unwired: 7 in, 4 out]
              }
            }
            n148 = local write "Init Complete"(w268) -> ()
            n149 = property on="Init Complete" class="Bool (strict)"("Val(Sgnl)"=w268) -> ()  [unwired: 2 in, 2 out]
            n150 = call "String_in_Reference.vi"("String"="Init. Complete") -> ()  [unwired: 18 in, 1 out]
          }
          frame Error {
          }
        }
      }
      frame "Wait for Purge" {
        # "Purge with control, or drawcount=0 or error,\nor stop, or \ndispense time - current draw time > purge guard time."
        n151 = local read "Dispense Times"() -> (w304:dbl[])
        n152 = local read "DrawCount"() -> (w305:i32)
        n153 = Index Array(array=w304, index=w305) -> (element=w302:dbl)
        n154 = local read "t*=0"() -> (w303:dbl)
        n155 = while {
          tunnel: w313 -> [w359]
          shift-right: [w350] -> w308
          shift-left: w306 -> [w349]
          tunnel: w312 -> [w352]
          tunnel: " Purge Condition. NextDispenseTime-Elaspse time < Purge Guard Time. t =   " ("string") -> [w331]
          tunnel: w303 -> [w326]
          tunnel: w302 -> [w325]
          tunnel: "Purge Guard Time(s)" -> [w324]
          i -> [w333]
          stop <- w335 stop-if-true
          n156 = local read "DrawCount"() -> (w345:i32)
          n157 = local read "Serial Data In"() -> (w323:string)
          n158 = local read "Use Agilent?"() -> (w321:bool)
          n159 = call "E-Time.vi"("error in (no error)"=w349) -> ("error out"=w348:errorcluster, "Elapsed Time (sec)"=w341:dbl)  [unwired: 8 in, 1 out]
          n160 = local read "Label Array"() -> (w322:string[])
          n161 = local read "Chanel List"() -> (w338:string)
          n162 = local read "Calibration File Array"() -> (w320:dbl[][])
          n163 = control-ref of="Tank Display"() -> (w351:refnum<vi>)
          n164 = Equal To 0?(x=w345) -> (x = 0?=w344:bool)
          n165 = Compound Arithmetic op=unknown(w325, w326, invert w324) -> (w330:dbl)
          n166 = call "Gather Test Data - Heatup Test new.vi"("Agilent Scan List"=w338, "Semiphore"=w359, "Equipment"=w352, "Tank Display Ref"=w351, "Agilent?"=w321, "Calibration Coefficients"=w320, "error in (no error)"=w348, "Serial Data In"=w323, "Agilent Label Array"=w322) -> ("Tc Tree"=w347:dbl[], "Output Data"=w339:string[][], "POWER"=w327:T4, "Voltage"=w332:dbl, "error out"=w350:errorcluster)  [unwired: 1 in, 1 out]
          "Tcs 1-6" <- w347
          n167 = local write "Voltage"(w332) -> ()
          n168 = Subtract(x=w325, y=w324) -> (x-y=w342:dbl)
          n169 = Number To Decimal String(number=w330) -> (decimal integer string=w329:string)  [unwired: 1 in]
          n170 = local write "Log Data"(w339) -> ()
          n171 = local write "POWER"(w327) -> ()
          n172 = Array To Cluster(array=w347) -> (cluster=w357:T22)
          n173 = Subtract(x=w341, y=w326) -> (x-y=w340:dbl)
          n174 = Build Array(w357) -> (→"Monitoring Temps Chart":T8)
          n175 = Greater?(x=w340, y=w342) -> (0:w337:bool)
          n176 = Number To Decimal String(number=w333) -> (decimal integer string=w353:string)  [unwired: 1 in]
          n177 = Equal To 0?(x=w333) -> (x = 0?=w334:bool)
          n178 = Unbundle By Name(w350) -> ("status"=w358:bool)
          n179 = local read "Stop Test Seqence"() -> (w328:bool)
          n180 = Concatenate Strings(w331, w329, w353, " Readings" ("string")) -> (w354:string)
          n181 = call "String_in_Reference.vi"("String"=w354) -> ()  [unwired: 18 in, 1 out]
          n182 = local read "T1"() -> (w346:u32)
          n183 = Compound Arithmetic op=OR(w328, w358, w337, "Purge Right Now", w344) -> (w335:bool)
          n184 = Compound Arithmetic op=OR(w334, w335) -> (w336:bool)
          n185 = case shown="True" w336 {
            tunnel: w339 -> [_ w361]
            frame False {
            }
            frame True {
              n186 = Index Array(array=w361, index (row)=1) -> (element=w360:string[])  [unwired: 1 in]
              n187 = local read "FileName"() -> (w365:path)
              n188 = call-poly <vilib>:"Write To Spreadsheet File.vi"("delimiter (\\t)"="," ("delimiter (\\t)"), "append to file? (new file:F)"=TRUE, "1D data"=w360, "file path (dialog if empty)"=w365) -> ()  [unwired: 4 in, 1 out]
            }
          }
          n189 = Wait (ms)(milliseconds to wait=w346) -> ()  [unwired: 1 out]
        }
        n190 = case shown="No Error" w308 {
          selector: w308 -> [w316 w319]
          tunnel: [w317 string[] ["Finish"] ("States")] -> w310
          tunnel: w311 -> [w317 _]
          tunnel: [w316 w319] -> w309
          frame No Error {
            # "Press it each time."
            n191 = local write "Purge Right Now"(FALSE ("Skip Waiting for Temp")) -> ()
          }
          frame Error {
          }
        }
      }
      frame "Purge" {
        n192 = flat-sequence {
          tunnel: [w401] -> w381
          tunnel: [w400] -> w380
          tunnel: [w405] -> w379
          frame #0 {
            n193 = local read "DrawCount"() -> (w399:i32)
            n194 = local read "DrawCount"() -> (w397:i32)
            n195 = local read "Temperature Schedule"() -> (w402:dbl[])
            n196 = local read "Flow Rate Schedule"() -> (w403:dbl[])
            n197 = Not Equal To 0?(x=w399) -> (x != 0?=w398:bool)
            n198 = case shown="True" w398 {
              tunnel: w397 -> [w406 w408]
              tunnel: [w406 w407] -> w396
              frame False {
              }
              frame True {
                n199 = Decrement(x=w408) -> (x-1=w407:i32)
              }
            }
            n200 = Index Array(array=w403, index=w396) -> (element=w401:dbl)
            n201 = Index Array(array=w402, index=w396) -> (element=w400:dbl)
            n202 = local write "Degrees F"(w400) -> ()
            n203 = local write "Flow Rate (GPM)"(w401) -> ()
            n204 = local read "Temp Band(+/- F)"() -> (w405:dbl)
            n205 = call "String_in_Reference.vi"("String"="PurgeBegins" ("string")) -> ()  [unwired: 18 in, 1 out]
          }
        }
        n206 = flat-sequence {
          tunnel: [TestedFlowratesScenarios."Build2,2B,Purge" ("Test Condition")] -> w374
          frame #0 {
            n207 = call "String_in_Reference.vi"("String"="Purge Sequence Start") -> ()  [unwired: 18 in, 1 out]
          }
        }
        n208 = control-ref of="Downspount Temp"() -> (w376:refnum<vi>)
        n209 = control-ref of="Downspount Flow"() -> (w389:refnum<vi>)
        n210 = call "Purge Water Sequence SM.vi"("Degree Setting"=w380, "Equipment"=w388, "Semiphore"=w367, "Flow rate setting"=w381, "Temp Band(+/- F)"=w379, "Error In"=w378, "Flow Chart Ref"=w389, "Temp Chart Ref"=w376, "Test Condition"=w374) -> ("Failed to Start Count"=w371:dbl, "Downspout Flow"=→"Downspout Flow":dbl, "Downspout Temp"=→"Downspout Temp":dbl, "Flow rate setting out"=→"Flow rate Adj":dbl, "Temp Setting Out"=→"TempAdj":dbl, "Error Out"=w373:errorcluster)  [unwired: 1 in]
        "Failed to Start Count" <- w371
        n211 = Greater Than 0?(x=w371) -> (x > 0?=w372:bool)
        n212 = case shown="True" w372 {
          tunnel: w373 -> [w414 w420]
          tunnel: [w414 w419] -> w366
          tunnel: w371 -> [_ w415]
          frame False {
          }
          frame True {
            n213 = local read "FileName"() -> (w421:path)
            n214 = Number To Decimal String(number=w415) -> (decimal integer string=w417:string)  [unwired: 1 in]
            n215 = Concatenate Strings("Failed to Start Count" ("string"), w417) -> (w416:string)
            n216 = call "Log String to Spreadsheet.vi"("String"=w416, "error in (no error)"=w420, "FileName"=w421) -> ("error out"=w419:errorcluster)  [unwired: 8 in]
          }
        }
        n217 = flat-sequence {
          tunnel: [w391] -> w369
          tunnel: w366 -> [w390]
          frame #0 {
            w393 = "PurgeComplete" ("string")
            n218 = local read "FileName"() -> (w392:path)
            n219 = call "Log String to Spreadsheet.vi"("String"=w393, "error in (no error)"=w390, "FileName"=w392) -> ("error out"=w391:errorcluster)  [unwired: 8 in]
            n220 = call "String_in_Reference.vi"("String"=w393) -> ()  [unwired: 18 in, 1 out]
          }
        }
        n221 = Unbundle By Name(w369) -> ("source"=w370:string)
        n222 = case shown="\"True\", Default" w370 {
          selector: w370 -> [_ w411]
          tunnel: w369 -> [w409 w412]
          tunnel: [w409 w410] -> w368
          frame "" {
          }
          frame "True", Default {
            # "Purge not stable case may\njust posts this warning."
            n223 = local read "FileName"() -> (w413:path)
            n224 = call "Log String to Spreadsheet.vi"("String"=w411, "error in (no error)"=w412, "FileName"=w413) -> ("error out"=w410:errorcluster)  [unwired: 8 in]
          }
        }
        n225 = case shown="Error" w368 {
          selector: w368 -> [w422 w425]
          tunnel: [w423 string[] ["Finish"] ("States")] -> w387
          tunnel: w385 -> [w423 _]
          tunnel: [w422 w425] -> w386
          frame No Error {
          }
          frame Error {
          }
        }
      }
      frame "Wait for Cutout" {
        # "At the end of the recovery period following\nthe first draw, record the maximum mean\ntank temperature observed after cut-out,\nT¯\nmax, 1, and the energy consumed by an electric\nresistance, gas or oil-fired water heater,\nQr. For heat pump water heaters, the total\nelectrical energy consumed during the first\nrecovery by the heat pump (including compressor,\nfan, controls, pump, etc.) and, if applicable,\nby the resistive element(s) shall be\nrecorded as Qr."
        n226 = local read "Chanel List"() -> (w437:string)
        n227 = while {
          tunnel: w440 -> [w472]
          shift-right: [w466] -> w430
          shift-left: w436 -> [w473]
          tunnel: w437 -> [w461]
          tunnel: [w451] -> w434
          tunnel: [w450] -> w427
          tunnel: [w449] -> w426
          i -> [w458]
          stop <- w457 continue-if-true
          # "Cutout for 2 samples in row"
          n228 = local read "Calibration File Array"() -> (w445:dbl[][])
          n229 = local read "Use Agilent?"() -> (w448:bool)
          n230 = local read "Serial Data In"() -> (w447:string)
          n231 = local read "Label Array"() -> (w446:string[])
          n232 = control-ref of="Tank Display"() -> (w463:refnum<vi>)
          n233 = local read "Equipment"() -> (w464:T1)
          n234 = call "Gather Test Data - Heatup Test new.vi"("Agilent Scan List"=w461, "Semiphore"=w472, "Equipment"=w464, "Tank Display Ref"=w463, "Agilent?"=w448, "Calibration Coefficients"=w445, "error in (no error)"=w473, "Serial Data In"=w447, "Agilent Label Array"=w446) -> ("Tc Tree"=w450:dbl[], "Output Data"=w462:string[][], "POWER"=w470:T4, "Voltage"=w456:dbl, "error out"=w466:errorcluster)  [unwired: 1 in, 1 out]
          "Tc Tree Check" <- w450
          n235 = Unbundle(w470) -> ("UE"=w467:bool, "LE"=w468:bool, "COMP"=w469:bool)  [unwired: 1 out]
          n236 = local write "POWER"(w470) -> ()
          n237 = local write "Log Data"(w462) -> ()
          n238 = Number To Decimal String(number=w458) -> (decimal integer string=w474:string)  [unwired: 1 in]
          n239 = Equal To 0?(x=w458) -> (x = 0?=w459:bool)
          n240 = Compound Arithmetic op=OR(w467, w468, w469) -> (w454:bool)
          n241 = local write "Voltage"(w456) -> ()
          n242 = local read "Stop Test Seqence"() -> (w455:bool)
          n243 = while {
            tunnel: w454 -> [w480]
            shift-right: [w481] -> w453
            shift-left: _ -> [w479]
            stop <- TRUE stop-if-true
            n244 = case shown="False" w480 {
              tunnel: [w484 0.0] -> w481
              tunnel: w479 -> [w483 _]
              frame False {
                n245 = Increment(x=w483) -> (x+1=w484:dbl)
              }
              frame True {
              }
            }
          }
          n246 = Concatenate Strings("WAIT FOR CUTOUT.  " ("String"), w474, " checks." ("string")) -> (w476:string)
          n247 = Unbundle By Name(w466) -> ("status"=w478:bool)
          n248 = call "String_in_Reference.vi"("String"=w476) -> ()  [unwired: 18 in, 1 out]
          n249 = Less Or Equal?(x=w453, y="Power Off Check Limit") -> (x <= y?=w451:bool)
          n250 = local read "T1"() -> (w471:u32)
          n251 = call-poly <vilib>:"Mean.vi"("X"=w450) -> ("mean"=w449:dbl)  [unwired: 1 out]
          "mean" <- w449
          n252 = Wait (ms)(milliseconds to wait=w471) -> ()  [unwired: 1 out]
          n253 = Compound Arithmetic op=AND(invert w478, w451, invert "Skip Waiting for Cutout", invert w455) -> (w457:bool)
          n254 = Compound Arithmetic op=OR(w459, invert w457) -> (w460:bool)
          n255 = case shown="True" w460 {
            tunnel: w462 -> [_ w486]
            frame False {
            }
            frame True {
              n256 = Index Array(array=w486, index (row)=1) -> (element=w487:string[])  [unwired: 1 in]
              n257 = local read "FileName"() -> (w491:path)
              n258 = call-poly <vilib>:"Write To Spreadsheet File.vi"("delimiter (\\t)"="," ("delimiter (\\t)"), "append to file? (new file:F)"=TRUE, "1D data"=w487, "file path (dialog if empty)"=w491) -> ()  [unwired: 4 in, 1 out]
            }
          }
        }
        n259 = Unbundle By Name(w430) -> ("status"=w429:bool)
        n260 = Select(t="Error" ("String"), s=w429, f="Skip" ("String")) -> (s? t:f=w432:string)
        n261 = local read "FileName"() -> (w439:path)
        n262 = Select(t=w432, s=w434, f="Cutout" ("String")) -> (s? t:f=w435:string)
        n263 = call "Log String to Spreadsheet.vi"("String"=w435, "error in (no error)"=w430, "FileName"=w439) -> ("error out"=w438:errorcluster)  [unwired: 8 in]
        n264 = case shown="No Error" w438 {
          selector: w438 -> [w493 w543]
          tunnel: [w496 string[] ["Finish"] ("States")] -> w444
          tunnel: w442 -> [w495 _]
          tunnel: [w494 w543] -> w443
          tunnel: w427 -> [w504 _]
          tunnel: w426 -> [w492 _]
          frame No Error {
            # "Press Each Time"
            n265 = local read "DrawCount"() -> (w501:i32)
            n266 = Index Array(array=w495, index=0) -> (element=w503:string)
            n267 = Equal?(x=w501, y=0) -> (x = y?=w498:bool)
            n268 = Equal?(x=w503, y="Wait for Next Draw") -> (x = y?=w499:bool)
            n269 = local write "Skip Waiting for Cutout"(FALSE ("Skip Waiting for Cutout")) -> ()
            n270 = And(x=w499, y=w498) -> (x .and. y?=w497:bool)
            n271 = case shown="True" w497 {
              tunnel: w504 -> [_ _]
              tunnel: [w508 w515] -> w496
              tunnel: w495 -> [w508 w514]
              tunnel: [w507 w511] -> w494
              tunnel: w493 -> [w507 w510]
              tunnel: w492 -> [_ w509]
              frame False {
              }
              frame True {
                n272 = local read "Temp Range Err"() -> (w512:bool)
                n273 = In Range and Coerce(upper limit="mean tank upper lim", x=w509, lower limit="meant tank lower lim") -> (In Range?=w516:bool)  [unwired: 1 out]
                n274 = case shown="False" w516 {
                  tunnel: [w523 w541] -> w515
                  tunnel: w514 -> [w524 w541]
                  tunnel: string[] ["Wait for Purge", "Purge", "Wait for Cutout", "Init Draw", "Term Draw0"] -> [w522 _]
                  tunnel: w512 -> [w521 _]
                  tunnel: [w520 w540] -> w511
                  tunnel: w510 -> [w519 w540]
                  frame False {
                    n275 = case shown="False" w521 {
                      tunnel: w524 -> [w532 _]
                      tunnel: [w531 string[] ["Finish"]] -> w523
                      tunnel: w522 -> [w530 _]
                      tunnel: [w527 w538] -> w520
                      tunnel: w519 -> [w528 w535]
                      frame False {
                        n276 = local read "FileName"() -> (w525:path)
                        n277 = Build Array (concatenate)(w530, w532) -> (w531:string[])
                        n278 = call "Log String to Spreadsheet.vi"("String"="Error: Mean Tank Temp", "error in (no error)"=w528, "FileName"=w525) -> ("error out"=w527:errorcluster)  [unwired: 8 in]
                        "Temp Range Err" <- TRUE ("Next Time Fail")
                      }
                      frame True {
                        n279 = local read "FileName"() -> (w533:path)
                        n280 = call "Log String to Spreadsheet.vi"("String"="Fail: Mean Tank Temp", "error in (no error)"=w535, "FileName"=w533) -> ("error out"=w534:errorcluster)  [unwired: 8 in]
                        n281 = call "Error Bool Enumerator.vi"("Error Enum"=HEWH_Error_Enumeration."Fail Mean Tank Temp", "Error In"=w534) -> ("Error Out"=w538:errorcluster)  [unwired: 7 in]
                      }
                    }
                  }
                  frame True {
                  }
                }
              }
            }
          }
          frame Error {
          }
        }
      }
      frame "Wait for Temp Decl" {
        n282 = local read "FileName"() -> (w545:path)
        n283 = Number To Fractional String(number="Temp Decline Hystersis") -> (F-format string=w549:string)  [unwired: 3 in]
        n284 = Concatenate Strings("Record each new Tave maximum.  Wating for Ave temp to decl by   " ("string"), w549, "degrees F." ("string")) -> (w544:string)
        n285 = call "Log String to Spreadsheet.vi"("String"=w544, "error in (no error)"=w547, "FileName"=w545) -> ("error out"=w546:errorcluster)  [unwired: 8 in]
        n286 = while {
          tunnel: w555 -> [w599]
          shift-right: [w588] -> w553
          shift-left: w546 -> [w598]
          tunnel: w554 -> [w589]
          shift-right: [w581] -> w552
          shift-left: _ -> [w585]
          tunnel: "Temp Decline Hystersis" -> [w572]
          i -> [w574]
          stop <- w573 stop-if-true
          n287 = local read "Calibration File Array"() -> (w565:dbl[][])
          n288 = local read "Serial Data In"() -> (w567:string)
          n289 = local read "Use Agilent?"() -> (w568:bool)
          n290 = local read "Label Array"() -> (w566:string[])
          n291 = control-ref of="Tank Display"() -> (w584:refnum<vi>)
          n292 = local read "Chanel List"() -> (w587:string)
          n293 = call "Gather Test Data - Heatup Test new.vi"("Agilent Scan List"=w587, "Semiphore"=w599, "Equipment"=w589, "Tank Display Ref"=w584, "Agilent?"=w568, "Calibration Coefficients"=w565, "error in (no error)"=w598, "Serial Data In"=w567, "Agilent Label Array"=w566) -> ("Tc Tree"=w594:dbl[], "Output Data"=w578:string[][], "POWER"=w577:T4, "Voltage"=w571:dbl, "error out"=w588:errorcluster)  [unwired: 1 in, 1 out]
          n294 = Number To Decimal String(number=w574) -> (decimal integer string=w591:string)  [unwired: 1 in]
          n295 = local write "Voltage"(w571) -> ()
          n296 = local write "POWER"(w577) -> ()
          n297 = call-poly <vilib>:"Mean.vi"("X"=w594) -> ("mean"=w582:dbl)  [unwired: 1 out]
          "T_Ave" <- w582
          n298 = local write "Log Data"(w578) -> ()
          n299 = Max & Min(x=w585, y=w582) -> (max(x,y)=w581:dbl)  [unwired: 1 out]
          "T_Ave_Max" <- w581
          n300 = Build Array (concatenate)(w594, w582) -> (w579:dbl[])
          "Tcs 1-6, Ave. 3" <- w579
          n301 = Subtract(x=w581, y=w582) -> (x-y=w586:dbl)
          n302 = Concatenate Strings("Wating for Ave temp to decl.  " ("string"), w591, " Readings." ("string")) -> (w592:string)
          n303 = Array To Cluster(array=w579) -> (cluster=w595:T23)
          n304 = call "String_in_Reference.vi"("String"=w592) -> ()  [unwired: 18 in, 1 out]
          n305 = Equal To 0?(x=w574) -> (x = 0?=w575:bool)
          n306 = Build Array(w595) -> (→"Temps Chart 2":T9)
          n307 = Greater Or Equal?(x=w586, y=w572) -> (x >= y?=w597:bool)
          n308 = local read "Stop Test Seqence"() -> (w570:bool)
          n309 = Unbundle By Name(w588) -> ("status"=w596:bool)
          n310 = local read "T1"() -> (w569:u32)
          n311 = Compound Arithmetic op=OR(w596, w597, "Skip Waiting for Temp 3", w570) -> (w573:bool)
          n312 = Compound Arithmetic op=OR(w575, w573) -> (w576:bool)
          n313 = case shown="True" w576 {
            tunnel: w578 -> [_ w600]
            frame False {
            }
            frame True {
              n314 = Index Array(array=w600, index (row)=1) -> (element=w601:string[])  [unwired: 1 in]
              n315 = local read "FileName"() -> (w605:path)
              n316 = call-poly <vilib>:"Write To Spreadsheet File.vi"("delimiter (\\t)"="," ("delimiter (\\t)"), "append to file? (new file:F)"=TRUE, "1D data"=w601, "file path (dialog if empty)"=w605) -> ()  [unwired: 4 in, 1 out]
            }
          }
          n317 = Wait (ms)(milliseconds to wait=w569) -> ()  [unwired: 1 out]
        }
        n318 = local read "FileName"() -> (w560:path)
        n319 = Number To Fractional String(number=w552) -> (F-format string=w556:string)  [unwired: 3 in]
        n320 = Concatenate Strings("Ave Temp Declined. Max Ave Tank Temp = " ("String"), w556) -> (w558:string)
        n321 = call "Log String to Spreadsheet.vi"("String"=w558, "error in (no error)"=w553, "FileName"=w560) -> ("error out"=w559:errorcluster)  [unwired: 8 in]
        n322 = case shown="No Error" w559 {
          selector: w559 -> [w606 w609]
          tunnel: [w607 string[] ["Finish"] ("States")] -> w564
          tunnel: w562 -> [w607 _]
          tunnel: [w606 w609] -> w563
          frame No Error {
          }
          frame Error {
          }
        }
      }
      frame "Init Draw" {
        # "Dont totalize flow on draw0"
        # "Valve must\nclose all the way\nbefore start works."
        n323 = flat-sequence {
          tunnel: [w639] -> w613
          tunnel: w612 -> [w639]
          frame #0 {
            n324 = local write "Drawing"(TRUE) -> ()
          }
        }
        n325 = local read "DrawCount"() -> (w621:i32)
        n326 = call "E-Time.vi"("error in (no error)"=w613) -> ("error out"=w627:errorcluster, "Elapsed Time (sec)"=w626:dbl)  [unwired: 8 in, 1 out]
        "Current Draw Start Time" <- w626
        n327 = local read "MW100"() -> (w611:refnum<visa-resource-name>)
        n328 = Equal?(x=1, y=w621) -> (x = y?=w629:bool)
        n329 = case shown="False" w629 {
          tunnel: w627 -> [w664 w673]
          tunnel: [w646 w671] -> w625
          tunnel: w626 -> [w665 _]
          tunnel: w617 -> [w663 _]
          tunnel: w611 -> [w662 _]
          tunnel: [w645 w672] -> w624
          frame True {
            n330 = local write "t*=0"(w665) -> ()
            n331 = call "YKMW100 Computation Control.vi"("VISA session"=w662, "Semiphore"=w663, "Mode"=T15."Reset Computation", "error in (no error)"=w664) -> ("error out"=w650:errorcluster)  [unwired: 10 in, 1 out]
            n332 = local read "Serial Data In"() -> (w643:string)
            n333 = local read "Use Agilent?"() -> (w644:bool)
            n334 = local read "Label Array"() -> (w642:string[])
            n335 = local read "Equipment"() -> (w648:T1)
            n336 = local read "Chanel List"() -> (w659:string)
            n337 = local read "Semiphore"() -> (w658:T2)
            n338 = control-ref of="Tank Display"() -> (w660:refnum<vi>)
            n339 = local read "Calibration File Array"() -> (w640:dbl[][])
            n340 = call "Gather Test Data - Heatup Test new.vi"("Agilent Scan List"=w659, "Semiphore"=w658, "Equipment"=w648, "Tank Display Ref"=w660, "Agilent?"=w644, "Calibration Coefficients"=w640, "error in (no error)"=w650, "Serial Data In"=w643, "Agilent Label Array"=w642) -> ("Output Data"=w645:string[][], "POWER"=w641:T4, "Voltage"=w649:dbl, "error out"=w647:errorcluster)  [unwired: 1 in, 2 out]
            n341 = local read "FileName"() -> (w652:path)
            n342 = local write "POWER"(w641) -> ()
            n343 = Index Array(array=w645, index (row)=1) -> (element=w655:string[])  [unwired: 1 in]
            n344 = local write "Voltage"(w649) -> ()
            n345 = call-poly <vilib>:"Write To Spreadsheet File.vi"("delimiter (\\t)"="," ("delimiter (\\t)"), "append to file? (new file:F)"=TRUE, "1D data"=w655, "file path (dialog if empty)"=w652) -> ("new file path (Not A Path if cancelled)"=w651:path)  [unwired: 4 in]
            n346 = call "Log String to Spreadsheet.vi"("String"="START (t*0)", "error in (no error)"=w647, "FileName"=w651) -> ("error out"=w646:errorcluster)  [unwired: 8 in]
          }
          frame False {
            n347 = local read "Serial Data In"() -> (w669:string)
            n348 = local read "Use Agilent?"() -> (w670:bool)
            n349 = local read "Label Array"() -> (w668:string[])
            n350 = local read "Equipment"() -> (w674:T1)
            n351 = local read "Chanel List"() -> (w682:string)
            n352 = local read "Semiphore"() -> (w681:T2)
            n353 = control-ref of="Tank Display"() -> (w683:refnum<vi>)
            n354 = local read "Calibration File Array"() -> (w666:dbl[][])
            n355 = call "Gather Test Data - Heatup Test new.vi"("Agilent Scan List"=w682, "Semiphore"=w681, "Equipment"=w674, "Tank Display Ref"=w683, "Agilent?"=w670, "Calibration Coefficients"=w666, "error in (no error)"=w673, "Serial Data In"=w669, "Agilent Label Array"=w668) -> ("Output Data"=w672:string[][], "POWER"=w667:T4, "Voltage"=w675:dbl, "error out"=w671:errorcluster)  [unwired: 1 in, 2 out]
            n356 = local write "Voltage"(w675) -> ()
            n357 = local write "POWER"(w667) -> ()
            n358 = local read "FileName"() -> (w676:path)
            n359 = Index Array(array=w672, index (row)=1) -> (element=w678:string[])  [unwired: 1 in]
            n360 = call-poly <vilib>:"Write To Spreadsheet File.vi"("delimiter (\\t)"="," ("delimiter (\\t)"), "append to file? (new file:F)"=TRUE, "1D data"=w678, "file path (dialog if empty)"=w676) -> ()  [unwired: 4 in, 1 out]
          }
        }
        n361 = local write "Log Data"(w624) -> ()
        n362 = call "Array_Search_For_Num.vi"("N Rows of Data"=w624, "Title?"="GALLONS") -> ("number"=→"M*-1":dbl)  [unwired: 12 in, 1 out]
        n363 = Number To Fractional String(number=w621) -> (F-format string=w630:string)  [unwired: 3 in]
        n364 = local read "FileName"() -> (w633:path)
        n365 = Concatenate Strings("Drawcount = " ("string"), w630) -> (w632:string)
        n366 = call "Log String to Spreadsheet.vi"("String"=w632, "error in (no error)"=w625, "FileName"=w633) -> ("error out"=w610:errorcluster)  [unwired: 8 in]
        n367 = local read "Expansion Tank?"() -> (w616:bool)
        n368 = Not Equal To 0?(x=w621) -> (x != 0?=w620:bool)
        n369 = call "HEWH Set Valves.vi"("VISA session"=w611, "Semiphore"=w617, "Expansion Tank?"=w616, "Valve Bank Setting"=ValveBankPositions."Draw", "Error In"=w610) -> ("dup VISA session"=w619:refnum<visa-resource-name>, "Error Out"=w618:errorcluster)  [unwired: 9 in]
        n370 = call "HEWH Totalize Flow Control.vi"("VISA session"=w619, "Semiphore"=w617, "Totalize Flow"=w620, "error in (no error)"=w618) -> ("error out"=w614:errorcluster)  [unwired: 10 in, 1 out]
        n371 = case shown="Error" w614 {
          selector: w614 -> [w684 w687]
          tunnel: [w685 string[] ["Finish"] ("States")] -> w635
          tunnel: w636 -> [w685 _]
          tunnel: [w684 w687] -> w634
          frame No Error {
          }
          frame Error {
          }
        }
      }
      frame "Term Draw0" {
        # "The draw may be terminated anytime after\ncut-in occurs."
        n372 = flat-sequence {
          tunnel: w697 -> [w702]
          tunnel: [w702] -> w694
          frame #0 {
            (unwired) T8 [] ("History Data")
          }
        }
        n373 = local read "FileName"() -> (w696:path)
        n374 = call "Log String to Spreadsheet.vi"("String"="Term Draw 0", "error in (no error)"=w694, "FileName"=w696) -> ("error out"=w692:errorcluster)  [unwired: 8 in]
        n375 = local read "Expansion Tank?"() -> (w690:bool)
        n376 = local read "MW100"() -> (w689:refnum<visa-resource-name>)
        n377 = call "HEWH Set Valves.vi"("VISA session"=w689, "Semiphore"=w688, "Expansion Tank?"=w690, "Valve Bank Setting"=ValveBankPositions."Heating", "Error In"=w692) -> ("Error Out"=w691:errorcluster)  [unwired: 9 in, 1 out]
        n378 = case shown="Error" w691 {
          selector: w691 -> [w703 w707]
          tunnel: [w704 string[] ["Finish"] ("States")] -> w700
          tunnel: w701 -> [w704 _]
          tunnel: [w703 w707] -> w699
          frame No Error {
          }
          frame Error {
            # "Press Each Time"
            n379 = local write "Skip Draw0"(FALSE ("Skip Draw0")) -> ()
          }
        }
      }
      frame "Wait for Next Draw" {
        # "When out of draws, waits for power off time, and turns off the power.  Then waits for finish time and finishes."
        # "Assumes Purging complete, and waiting on Time trigger."
        n380 = local read "Dispense Schedule"() -> (w711:dbl[])
        n381 = local read "DrawCount"() -> (w709:i32)
        n382 = Array Size(array=w711) -> (size(s)=w708:i32)
        n383 = Greater?(x=w708, y=w709) -> (0:w710:bool)
        n384 = case shown="False" w710 {
          tunnel: w713 -> [w723 _]
          tunnel: [w722 w854] -> w716
          tunnel: w712 -> [w719 w848]
          tunnel: [w724 w855] -> w714
          tunnel: w708 -> [_ w850]
          frame False {
            w717 = "Wait for Test Complete" ("String")
            n385 = local read "FileName"() -> (w720:path)
            n386 = local read "PowerON"() -> (w721:bool)
            n387 = call "Log String to Spreadsheet.vi"("String"=w717, "error in (no error)"=w719, "FileName"=w720) -> ("error out"=w718:errorcluster)  [unwired: 8 in]
            n388 = call "String_in_Reference.vi"("String"=w717) -> ()  [unwired: 18 in, 1 out]
            n389 = case shown="True" w721 {
              tunnel: [string[] ["Finish"] ("States") string[] ["Wait for Next Draw"] ("States")] -> w724
              tunnel: w718 -> [w755 w790]
              tunnel: w723 -> [w749 _]
              tunnel: [w732 w788] -> w722
              frame False {
                # "At 24 hours, record the\nmean tank temperature, T¯ 24, and the electric\nand/or fuel instrument readings."
                n390 = while {
                  tunnel: w755 -> [w765]
                  tunnel: [w764] -> w750
                  stop <- w758 stop-if-true
                  # "Wait for Finish Time."
                  n391 = local read "End Log Duration"() -> (w762:dbl)
                  n392 = local read "Power Off Time"() -> (w763:dbl)
                  n393 = local read "Stop Test Seqence"() -> (w757:bool)
                  n394 = local read "t*=0"() -> (w766:dbl)
                  n395 = call "E-Time.vi"("error in (no error)"=w765) -> ("error out"=w764:errorcluster, "Elapsed Time (sec)"=w768:dbl)  [unwired: 8 in, 1 out]
                  n396 = local read "T1"() -> (w760:u32)
                  n397 = Add(x=w762, y=w763) -> (x+y=w761:dbl)
                  n398 = Subtract(x=w768, y=w766) -> (x-y=w767:dbl)
                  n399 = Greater Or Equal?(x=w767, y=w761) -> (x >= y?=w759:bool)
                  n400 = Or(x=w759, y=w757) -> (x .or. y?=w758:bool)
                  n401 = Wait (ms)(milliseconds to wait=w760) -> ()  [unwired: 1 out]
                }
                n402 = local read "Calibration File Array"() -> (w725:dbl[][])
                n403 = local read "Serial Data In"() -> (w727:string)
                n404 = local read "Use Agilent?"() -> (w728:bool)
                n405 = local read "Label Array"() -> (w726:string[])
                n406 = local read "Chanel List"() -> (w734:string)
                n407 = local read "Equipment"() -> (w752:T1)
                n408 = control-ref of="Tank Display"() -> (w751:refnum<vi>)
                n409 = call "Gather Test Data - Heatup Test new.vi"("Agilent Scan List"=w734, "Semiphore"=w749, "Equipment"=w752, "Tank Display Ref"=w751, "Agilent?"=w728, "Calibration Coefficients"=w725, "error in (no error)"=w750, "Serial Data In"=w727, "Agilent Label Array"=w726) -> ("Tc Tree"=w747:dbl[], "Output Data"=w737:string[][], "POWER"=w735:T4, "PowerData"=w748:T24, "Voltage"=w729:dbl, "error out"=w739:errorcluster)  [unwired: 1 in]
                n410 = Unbundle By Name(w748) -> ("WattHours"=w741:dbl)
                n411 = local write "Voltage"(w729) -> ()
                n412 = call-poly <vilib>:"Mean.vi"("X"=w747) -> ("mean"=w746:dbl)  [unwired: 1 out]
                n413 = local write "POWER"(w735) -> ()
                n414 = Index Array(array=w737, index (row)=1) -> (element=w736:string[])  [unwired: 1 in]
                n415 = Number To Decimal String(number=w746) -> (decimal integer string=w745:string)  [unwired: 1 in]
                n416 = Number To Decimal String(number=w741) -> (decimal integer string=w740:string)  [unwired: 1 in]
                n417 = local read "FileName"() -> (w730:path)
                n418 = local write "Log Data"(w737) -> ()
                n419 = call-poly <vilib>:"Write To Spreadsheet File.vi"("delimiter (\\t)"="," ("delimiter (\\t)"), "append to file? (new file:F)"=TRUE, "1D data"=w736, "file path (dialog if empty)"=w730) -> ()  [unwired: 4 in, 1 out]
                n420 = Concatenate Strings("Measured at Tfinal: Tank Ave Temp = " ("String"), w745, ", Watts Hours = " ("String"), w740) -> (w743:string)
                n421 = call "Log String to Spreadsheet.vi"("String"=w743, "error in (no error)"=w739, "FileName"=w730) -> ("error out"=w733:errorcluster)  [unwired: 8 in]
                n422 = call "Log String to Spreadsheet.vi"("String"="Test Complete", "error in (no error)"=w733, "FileName"=w730) -> ("error out"=w732:errorcluster)  [unwired: 8 in]
              }
              frame True {
                w796 = T25 30 items=["4-20_OUT", "Pres_HI1", "Pres_HI2", "Pres_LOW", "Pres_PIN", "HEATER_TOP", "HEATER_BOT", "T_Shell", "FLOWMETER", "WATT_SENSE", "WH_TICK", "Tc_1", "Tc_2", "Tc_3", "Tc_4", "Tc_5", "Tc_6", "Tc_down", "T_Shell_2", "T_Shell_3", "T_Shell_4", "RTD_IN", "RTD_OUT", "RTD_AMB", "INTF_TEMPFLO", "INTF_READY", "INTF_START", "INTF_STOP", "DRM_LOW", "DRM_HIGH", "PWR_MAIN", "VLV_DUMP", "VLV_OUT", "VLV_IN", "WATT_HOURS", "FLOW(SAMPLE)", "GALLONS", "FLOW(GPM)"] ("Channel_Enum")
                # "Delay Long enough for last \nserial communication data acq to \ncomplete then Turn Off Power"
                n423 = local read "FileName"() -> (w800:path)
                n424 = call "Log String to Spreadsheet.vi"("String"="Wait for final Cutoff", "error in (no error)"=w790, "FileName"=w800) -> ("error out"=w801:errorcluster)  [unwired: 8 in]
                n425 = while {
                  tunnel: "Power Off Guard Time20s)" -> [w812]
                  shift-right: [w814] -> w789
                  shift-left: w801 -> [w819]
                  stop <- w807 stop-if-true
                  n426 = local read "Power Off Time"() -> (w813:dbl)
                  n427 = call "E-Time.vi"("error in (no error)"=w819) -> ("error out"=w814:errorcluster, "Elapsed Time (sec)"=w817:dbl)  [unwired: 8 in, 1 out]
                  n428 = local read "t*=0"() -> (w816:dbl)
                  n429 = local read "Stop Test Seqence"() -> (w809:bool)
                  n430 = call "String_in_Reference.vi"("String"="Wait for power off Time.") -> ()  [unwired: 18 in, 1 out]
                  n431 = local read "T1"() -> (w815:u32)
                  n432 = Subtract(x=w817, y=w816) -> (x-y=w818:dbl)
                  n433 = Subtract(x=w813, y=w812) -> (x-y=w811:dbl)
                  n434 = Wait (ms)(milliseconds to wait=w815) -> ()  [unwired: 1 out]
                  n435 = Greater?(x=w818, y=w811) -> (0:w808:bool)
                  n436 = Compound Arithmetic op=OR(w808, w809) -> (w807:bool)
                }
                n437 = local read "Chanel List"() -> (w782:string)
                n438 = local read "Semiphore"() -> (w799:T2)
                n439 = expression code="1000*x"("Power Off Guard Time20s)") -> (w776:u32)
                n440 = while {
                  tunnel: w799 -> [w837]
                  tunnel: w782 -> [w831]
                  tunnel: w789 -> [w835]
                  tunnel: [w834] -> w779
                  i -> [w827]
                  stop <- w826 continue-if-true
                  n441 = local read "Calibration File Array"() -> (w820:dbl[][])
                  n442 = local read "Use Agilent?"() -> (w823:bool)
                  n443 = local read "Serial Data In"() -> (w822:string)
                  n444 = local read "Label Array"() -> (w821:string[])
                  n445 = control-ref of="Tank Display"() -> (w830:refnum<vi>)
                  n446 = local read "Equipment"() -> (w838:T1)
                  n447 = local read "T1"() -> (w836:u32)
                  n448 = call "Gather Test Data - Heatup Test new.vi"("Agilent Scan List"=w831, "Semiphore"=w837, "Equipment"=w838, "Tank Display Ref"=w830, "Agilent?"=w823, "Calibration Coefficients"=w820, "error in (no error)"=w835, "Serial Data In"=w822, "Agilent Label Array"=w821) -> ("Output Data"=w833:string[][], "POWER"=w832:T4, "Voltage"=w825:dbl, "error out"=w834:errorcluster)  [unwired: 1 in, 2 out]
                  n449 = Equal To 0?(x=w827) -> (x = 0?=w828:bool)
                  n450 = Wait (ms)(milliseconds to wait=w836) -> ()  [unwired: 1 out]
                  n451 = local read "Stop Test Seqence"() -> (w824:bool)
                  n452 = Unbundle(w832) -> ("UE"=w841:bool, "LE"=w840:bool, "COMP"=w839:bool)  [unwired: 1 out]
                  n453 = local write "Log Data"(w833) -> ()
                  n454 = local write "POWER"(w832) -> ()
                  n455 = Compound Arithmetic op=OR(w841, w840, w839, w824) -> (w826:bool)
                  n456 = Or(x=w828, y=w826) -> (x .or. y?=w829:bool)
                  n457 = case shown="True" w829 {
                    tunnel: w833 -> [_ w842]
                    frame False {
                    }
                    frame True {
                      n458 = Index Array(array=w842, index (row)=1) -> (element=w843:string[])  [unwired: 1 in]
                      n459 = local read "FileName"() -> (w845:path)
                      n460 = call-poly <vilib>:"Write To Spreadsheet File.vi"("delimiter (\\t)"="," ("delimiter (\\t)"), "append to file? (new file:F)"=TRUE, "1D data"=w843, "file path (dialog if empty)"=w845) -> ()  [unwired: 4 in, 1 out]
                    }
                  }
                  n461 = local write "Voltage"(w825) -> ()
                }
                n462 = flat-sequence {
                  tunnel: w779 -> [w806]
                  tunnel: [w805] -> w777
                  frame #0 {
                    n463 = local read "FileName"() -> (w802:path)
                    n464 = local write "PowerON"(FALSE ("PowerON")) -> ()
                    n465 = call "Log String to Spreadsheet.vi"("String"="Power Off", "error in (no error)"=w806, "FileName"=w802) -> ("error out"=w805:errorcluster)  [unwired: 8 in]
                  }
                }
                n466 = local read "Chanel List"() -> (w781:string)
                n467 = local read "MW100"() -> (w791:refnum<visa-resource-name>)
                n468 = local read "Serial Data In"() -> (w771:string)
                n469 = control-ref of="Tank Display"() -> (w798:refnum<vi>)
                n470 = local read "Use Agilent?"() -> (w772:bool)
                n471 = local read "Label Array"() -> (w770:string[])
                n472 = call "Delay mS.vi"("Error In"=w777, "milliseconds to wait"=w776) -> ("Error Out"=w778:errorcluster)  [unwired: 13 in]
                n473 = call "Generic - DO1.vi"("VISA session"=w791, "Semiphore"=w799, "Channel_Enum"=w796, "Relay Status (0:CLOSED)"=enum8{"CLOSED", "OPEN"}."CLOSED", "Error In"=w778) -> ("error out"=w780:errorcluster)  [unwired: 9 in, 1 out]
                n474 = local read "Calibration File Array"() -> (w769:dbl[][])
                n475 = local read "Equipment"() -> (w797:T1)
                n476 = call "Gather Test Data - Heatup Test new.vi"("Agilent Scan List"=w781, "Semiphore"=w799, "Equipment"=w797, "Tank Display Ref"=w798, "Agilent?"=w772, "Calibration Coefficients"=w769, "error in (no error)"=w780, "Serial Data In"=w771, "Agilent Label Array"=w770) -> ("Output Data"=w785:string[][], "POWER"=w783:T4, "Voltage"=w774:dbl, "error out"=w788:errorcluster)  [unwired: 1 in, 2 out]
                n477 = local write "Voltage"(w774) -> ()
                n478 = Index Array(array=w785, index (row)=1) -> (element=w784:string[])  [unwired: 1 in]
                n479 = local write "POWER"(w783) -> ()
                n480 = local write "Log Data"(w785) -> ()
                n481 = local read "FileName"() -> (w794:path)
                n482 = call-poly <vilib>:"Write To Spreadsheet File.vi"("delimiter (\\t)"="," ("delimiter (\\t)"), "append to file? (new file:F)"=TRUE, "1D data"=w784, "file path (dialog if empty)"=w794) -> ()  [unwired: 4 in, 1 out]
              }
            }
          }
          frame True {
            (unwired) string[] ["Init Draw", "Draw", "Term Draw", "Wait for Cutout", "Wait for Temp Decl", "Wait for Purge", "Purge", "Wait for Next Draw"]  # First Draw States SE
            # "3 cases.  First Draw, Need Max temp.\nIntermediate draws don't and might not cutoff.\nLast draw won't wait for a purge condition and need\nmax temp."
            n483 = while {
              shift-right: [w879] -> w852
              shift-left: w848 -> [w872]
              tunnel: [w868] -> _
              i -> [w876]
              stop <- w869 stop-if-true
              n484 = local read "Dispense Times"() -> (w871:dbl[])
              n485 = local read "DrawCount"() -> (w870:i32)
              n486 = Number To Decimal String(number=w876) -> (decimal integer string=w862:string)  [unwired: 1 in]
              n487 = local read "t*=0"() -> (w865:dbl)
              n488 = call "E-Time.vi"("error in (no error)"=w872) -> ("error out"=w879:errorcluster, "Elapsed Time (sec)"=w874:dbl)  [unwired: 8 in, 1 out]
              n489 = local read "T1"() -> (w873:u32)
              n490 = Index Array(array=w871, index=w870) -> (element=w866:dbl)
              n491 = Add(x=w865, y=w866) -> (x+y=w860:dbl)
              n492 = Subtract(x=w874, y=w865) -> (x-y=w875:dbl)
              n493 = Unbundle By Name(w872) -> ("status"=w867:bool)
              n494 = local read "Stop Test Seqence"() -> (w859:bool)
              n495 = Number To Fractional String(number=w860) -> (F-format string=w864:string)  [unwired: 3 in]
              n496 = Greater Or Equal?(x=w875, y=w866) -> (x >= y?=w868:bool)
              n497 = Concatenate Strings("WAIT FOR T=" ("String"), w864, ".  ", w862, " checks." ("string")) -> (w878:string)
              n498 = Wait (ms)(milliseconds to wait=w873) -> ()  [unwired: 1 out]
              n499 = call "String_in_Reference.vi"("String"=w878) -> ()  [unwired: 18 in, 1 out]
              n500 = Compound Arithmetic op=OR(w868, w867, w859) -> (w869:bool)
            }
            n501 = flat-sequence {
              tunnel: [w857] -> w853
              tunnel: w852 -> [w857]
              tunnel: [w856] -> w849
              frame #0 {
                n502 = local read "DrawCount"() -> (w858:i32)
                n503 = Increment(x=w858) -> (x+1=w856:i32)
                n504 = local write "DrawCount"(w856) -> ()
              }
            }
            n505 = Equal?(x=w849, y=w850) -> (x = y?=w851:bool)
            n506 = case shown="False" w851 {
              tunnel: [w884 w887] -> w855
              tunnel: [w883 w888] -> w854
              tunnel: w853 -> [w883 w888]
              tunnel: w849 -> [w881 _]
              frame False {
                n507 = Equal?(x=w881, y=1) -> (x = y?=w882:bool)
                n508 = case shown="False" w882 {
                  tunnel: [w885 w886] -> w884
                  frame False {
                    w885 = string[] ["Init Draw", "Draw", "Term Draw", "Wait for Purge", "Purge", "Wait for Next Draw"]  # Draw States
                    # "Intermediate Draws"
                  }
                  frame True {
                    w886 = string[] ["Init Draw", "Draw", "Term Draw", "Wait for Purge", "Purge", "Wait for Next Draw"]  # First Draw States
                    # "First Draw"
                  }
                }
              }
              frame True {
                w887 = string[] ["Init Draw", "Draw", "Term Draw", "Wait for Cutout", "Wait for Temp Decl", "Wait for Next Draw"]  # Last Draw States
                w889 = TRUE ("Special Last Draw")
                # "Last Draws"
                n509 = local write "Special Last Draw"(w889) -> ()
                "LastDraw" <- w889
              }
            }
          }
        }
      }
      frame "Draw" {
        n510 = flat-sequence {
          tunnel: [w909] -> w895
          tunnel: w894 -> [w909]
          frame #0 {
            "Drawing" <- TRUE
          }
        }
        n511 = while {
          shift-right: [w920] -> w891
          shift-left: w895 -> [w944]
          tunnel: w901 -> [w935]
          tunnel: [w935] -> w897
          shift-right: [w954] -> _
          shift-left: 15.0 ("GPM") -> [w953]
          shift-right: [w940] -> _
          shift-left: 0.0 ("GPM") -> [w941]
          tunnel: w896 -> [_]
          stop <- w956 stop-if-true
          # "T*max is max outlet temp."
          # "Sum of Temperatures"
          # "time to read"
          # "Start Special Case Immediately.  If after 30 sec, T< last\ntime, stop and discard measuremnts."
          # "(For Last Draw, If after 30 sec, T< last tmin, stop and discard measurements, else continue)"
          # "Record output water temp after 15 secs, and at 5 sec intervals thereafter\nMonitor inlet water temp, must be 58 +/- 2 F\nTerminate draw when output temp = T*max -25F, record T*min"
          n512 = local read "Current Draw Start Time"() -> (w951:dbl)
          n513 = local read "Label Array"() -> (w939:string[])
          n514 = call "E-Time.vi"("error in (no error)"=w944) -> ("error out"=w937:errorcluster, "Elapsed Time (sec)"=w917:dbl)  [unwired: 8 in, 1 out]
          n515 = stacked-sequence {
            seq-local: [w958 _ _ _ _] -> [_ w973 w977 w985 w991]
            tunnel: [_ w975 _ _ _] -> w921
            tunnel: w937 -> [w969 _ _ _ _]
            tunnel: [_ _ w978 _ _] -> w932
            tunnel: [w968 _ _ _ _] -> w936
            tunnel: w935 -> [w965 _ _ _ _]
            tunnel: [_ _ _ _ w989] -> w918
            tunnel: [_ w972 _ _ _] -> w923
            tunnel: w939 -> [w959 _ _ _ _]
            tunnel: [w958 _ _ _ _] -> w938
            tunnel: w917 -> [_ w971 _ w981 _]
            frame #0 {
              n516 = local read "Serial Data In"() -> (w960:string)
              n517 = local read "Equipment"() -> (w962:T1)
              n518 = control-ref of="Tank Display"() -> (w964:refnum<vi>)
              n519 = local read "Chanel List"() -> (w966:string)
              n520 = local read "Calibration File Array"() -> (w957:dbl[][])
              n521 = call "Gather Test Data - Heatup Test new.vi"("Agilent Scan List"=w966, "Semiphore"=w965, "Equipment"=w962, "Tank Display Ref"=w964, "Agilent?"=FALSE, "Calibration Coefficients"=w957, "error in (no error)"=w969, "Serial Data In"=w960, "Agilent Label Array"=w959) -> ("Output Data"=w958:string[][], "POWER"=w967:T4, "Voltage"=w963:dbl, "error out"=w968:errorcluster)  [unwired: 1 in, 2 out]
              n522 = local write "POWER"(w967) -> ()
              n523 = local write "Voltage"(w963) -> ()
            }
            frame #1 {
              # "Tmin assumed to\nbe last TOUT"
              n524 = local write "Log Data"(w973) -> ()
              n525 = call "Array_Search_For_Num.vi"("N Rows of Data"=w973, "Title?"="FLOW(GPM)" ("String")) -> ("number"=w972:dbl)  [unwired: 12 in, 1 out]
              n526 = call "Chart - Buffer Data.vi"("Time"=w971, "Data"=w972) -> ("XY chart data"=→"Flowmeter":cluster{"x":dbl, "y":dbl}[])  [unwired: 9 in]
              n527 = local read "Tank Display"() -> (w976:T5)
              n528 = Unbundle By Name(w976) -> ("TOUT"=w975:dbl)
            }
            frame #2 {
              n529 = call "Array_Search_For_Num.vi"("N Rows of Data"=w977, "Title?"="GALLONS") -> ("number"=w978:dbl)  [unwired: 12 in, 1 out]
            }
            frame #3 {
              n530 = local read "T*min"() -> (w983:dbl)
              n531 = call "Array_Search_For_Num.vi"("N Rows of Data"=w985, "Title?"="RTD_OUT" ("String")) -> ("number"=w982:dbl)  [unwired: 12 in, 1 out]
              n532 = local read "T*Max"() -> (w986:dbl)
              n533 = Max & Min(x=w986, y=w982) -> (max(x,y)=w987:dbl)  [unwired: 1 out]
              n534 = call "Chart - Buffer Data.vi"("Time"=w981, "Data"=w982) -> ("XY chart data"=→"RTD Out":cluster{"x":dbl, "y":dbl}[])  [unwired: 9 in]
              n535 = Max & Min(x=w982, y=w983) -> (min(x,y)=w984:dbl)  [unwired: 1 out]
              n536 = local write "T*Max"(w987) -> ()
              n537 = local write "T*min"(w984) -> ()
            }
            frame #4 {
              n538 = call "Array_Search_For_Num.vi"("N Rows of Data"=w991, "Title?"="Tc_down" ("String")) -> ("number"=w989:dbl)  [unwired: 12 in, 1 out]
              "TcDown" <- w989
            }
          }
          n539 = Subtract(x=w917, y=w951) -> (x-y=w927:dbl)
          n540 = Greater Or Equal?(x=w927, y=w953) -> (x >= y?=w942:bool)
          n541 = case shown="True" w942 {
            tunnel: [w993 w1015] -> w954
            tunnel: w953 -> [w993 w1014]
            tunnel: w936 -> [w994 w998]
            tunnel: [w996 w1013] -> w940
            tunnel: w941 -> [w996 w1012]
            tunnel: [FALSE w1011] -> w952
            tunnel: [w992 w1010] -> w926
            tunnel: [w994 w998] -> w943
            tunnel: w938 -> [_ w1000]
            tunnel: w932 -> [_ w999]
            tunnel: w921 -> [_ w997]
            frame False {
              n542 = local read "Gal Target"() -> (w992:dbl)
            }
            frame True {
              n543 = local read "LastDraw"() -> (w1006:bool)
              n544 = Add(x=5.0, y=w1014) -> (x+y=w1015:dbl)
              n545 = local read "FileName"() -> (w1003:path)
              n546 = Index Array(array=w1000, index (row)=1) -> (element=w1001:string[])  [unwired: 1 in]
              n547 = call-poly <vilib>:"Write To Spreadsheet File.vi"("delimiter (\\t)"="," ("delimiter (\\t)"), "append to file? (new file:F)"=TRUE, "1D data"=w1001, "file path (dialog if empty)"=w1003) -> ()  [unwired: 4 in, 1 out]
              n548 = case shown="True" w1006 {
                tunnel: w999 -> [_ w1024]
                tunnel: w999 -> [w1021 _]
                tunnel: [w1020 w1026] -> w1011
                tunnel: [w1016 w1023] -> w1010
                frame False {
                  n549 = local read "DrawCount"() -> (w1019:i32)
                  n550 = local read "Dispense Schedule"() -> (w1022:dbl[])
                  n551 = Delete From Array(array=w1022, length=w1019, index=0) -> (deleted portion=w1017:dbl[])  [unwired: 1 out]
                  n552 = Add Array Elements(numeric array=w1017) -> (sum=w1016:dbl)
                  n553 = Greater Or Equal?(x=w1021, y=w1016) -> (x >= y?=w1020:bool)
                }
                frame True {
                  n554 = local read "Dispense Schedule"() -> (w1027:dbl[])
                  n555 = Add Array Elements(numeric array=w1027) -> (sum=w1025:dbl)
                  n556 = Greater Or Equal?(x=w1024, y=w1025) -> (x >= y?=w1026:bool)
                  n557 = Subtract(x=w1025, y=w1024) -> (x-y=w1023:dbl)
                }
              }
              n558 = Add(x=w1012, y=w997) -> (x+y=w1013:dbl)
              n559 = expression code="x/5-3"(w1015) -> (w1008:dbl)
              n560 = Divide(x=w1013, y=w1008) -> (x/y=→"T*Ave":dbl)
              "Volume(Gal.)" <- w999
            }
          }
          "Gal Target" <- w926
          n561 = To Long Integer(number=w926) -> (32bit integer=w922:i32)
          n562 = local read "TempAdj"() -> (w919:dbl)
          n563 = Number To Decimal String(number=w922) -> (decimal integer string=w948:string)  [unwired: 1 in]
          n564 = local read "MW100"() -> (w934:refnum<visa-resource-name>)
          n565 = Concatenate Strings("Draw until " ("string"), w948, "gallons." ("string")) -> (w946:string)
          n566 = call "String_in_Reference.vi"("String"=w946) -> ()  [unwired: 18 in, 1 out]
          n567 = local read "DrawCount"() -> (w911:i32)
          n568 = local read "Temperature Schedule"() -> (w915:dbl[])
          n569 = local read "Flow Rate Schedule"() -> (w916:dbl[])
          n570 = Decrement(x=w911) -> (x-1=w912:i32)
          n571 = local read "Stop Test Seqence"() -> (w945:bool)
          n572 = Index Array(array=w915, index=w912) -> (element=w913:dbl)
          n573 = Subtract(x=w913, y="RTDin to Downspout Offset") -> (x-y=w924:dbl)
          n574 = Index Array(array=w916, index=w912) -> (element=w914:dbl)
          n575 = call "HEWH Flow and Temp Adjustment.vi"("MW100"=w934, "FlowReading"=w923, "Flow In"="Flow Adj", "K(0.1)"="K(0.1)", "TempReading"=w918, "Error In"=w943, "FlowTarget"=w914, "Temp Target"=w924, "Temp In"=w919, "Semiphore"=w935, "Elapsed Time (sec)"=w927, "Flow Adjust Time (3s)"="Adj Time") -> ("Flow Out"=w929:dbl, "Temp Out"=w931:dbl, "Error Out"=w920:errorcluster)  [unwired: 5 in]
          n576 = Unbundle By Name(w920) -> ("status"=w955:bool)
          n577 = local write "TempAdj"(w931) -> ()
          n578 = local write "Flow Adj"(w929) -> ()
          n579 = local read "T5"() -> (w950:u32)
          n580 = Compound Arithmetic op=OR(w955, w952, w945) -> (w956:bool)
          n581 = Wait (ms)(milliseconds to wait=w950) -> ()  [unwired: 1 out]
        }
        n582 = case shown="Error" w891 {
          selector: w891 -> [w902 w908]
          tunnel: [w904 string[] ["Finish"] ("States")] -> w892
          tunnel: w893 -> [w904 _]
          tunnel: [w903 w908] -> w890
          frame No Error {
            n583 = flat-sequence {
              tunnel: [w906] -> w903
              tunnel: w902 -> [w906]
              frame #0 {
                n584 = local write "Drawing"(FALSE) -> ()
              }
            }
          }
          frame Error {
          }
        }
      }
      frame "Draw0" {
        n585 = local read "Flow Adj"() -> (w1028:dbl)
        n586 = while {
          shift-right: [w1063] -> w1034
          shift-left: w1031 -> [w1064]
          shift-right: [w1066] -> _
          shift-left: w1028 -> [w1070]
          tunnel: w1035 -> [w1065]
          tunnel: [w1065] -> w1030
          tunnel: w1029 -> [_]
          stop <- w1071 stop-if-true
          # "Draw until power for heating kicks on."
          n587 = call "E-Time.vi"("error in (no error)"=w1064) -> ("error out"=w1068:errorcluster, "Elapsed Time (sec)"=w1041:dbl)  [unwired: 8 in, 1 out]
          n588 = local read "Label Array"() -> (w1047:string[])
          n589 = stacked-sequence {
            seq-local: [w1095 _ _ _] -> [_ w1106 w1111 w1115]
            tunnel: w1068 -> [w1097 _ _ _]
            tunnel: [w1096 _ _ _] -> w1056
            tunnel: w1065 -> [w1093 _ _ _]
            tunnel: [_ _ _ w1113] -> w1049
            tunnel: [_ w1104 _ _] -> w1048
            tunnel: w1047 -> [w1087 _ _ _]
            tunnel: [w1086 _ _ _] -> w1042
            tunnel: w1041 -> [_ w1103 w1108 _]
            frame #0 {
              n590 = local read "Serial Data In"() -> (w1088:string)
              n591 = local read "Equipment"() -> (w1090:T1)
              n592 = control-ref of="Tank Display"() -> (w1092:refnum<vi>)
              n593 = local read "Chanel List"() -> (w1094:string)
              n594 = local read "Calibration File Array"() -> (w1085:dbl[][])
              n595 = call "Gather Test Data - Heatup Test new.vi"("Agilent Scan List"=w1094, "Semiphore"=w1093, "Equipment"=w1090, "Tank Display Ref"=w1092, "Agilent?"=FALSE, "Calibration Coefficients"=w1085, "error in (no error)"=w1097, "Serial Data In"=w1088, "Agilent Label Array"=w1087) -> ("Output Data"=w1095:string[][], "POWER"=w1086:T4, "Voltage"=w1091:dbl, "error out"=w1096:errorcluster)  [unwired: 1 in, 2 out]
              n596 = local write "POWER"(w1086) -> ()
              n597 = local write "Voltage"(w1091) -> ()
              n598 = local read "FileName"() -> (w1100:path)
              n599 = Index Array(array=w1095, index (row)=1) -> (element=w1102:string[])  [unwired: 1 in]
              n600 = call-poly <vilib>:"Write To Spreadsheet File.vi"("delimiter (\\t)"="," ("delimiter (\\t)"), "append to file? (new file:F)"=TRUE, "1D data"=w1102, "file path (dialog if empty)"=w1100) -> ()  [unwired: 4 in, 1 out]
            }
            frame #1 {
              # "Tmin assumed to\nbe last TOUT"
              n601 = local write "Log Data"(w1106) -> ()
              n602 = call "Array_Search_For_Num.vi"("N Rows of Data"=w1106, "Title?"="FLOW(GPM)" ("String")) -> ("number"=w1104:dbl)  [unwired: 12 in, 1 out]
              n603 = call "Chart - Buffer Data.vi"("Time"=w1103, "Data"=w1104) -> ("XY chart data"=→"FlowMeter During Draw0":cluster{"x":dbl, "y":dbl}[])  [unwired: 9 in]
            }
            frame #2 {
              n604 = call "Array_Search_For_Num.vi"("N Rows of Data"=w1111, "Title?"="RTD_OUT" ("String")) -> ("number"=w1109:dbl)  [unwired: 12 in, 1 out]
              n605 = call "Chart - Buffer Data.vi"("Time"=w1108, "Data"=w1109) -> ("XY chart data"=→"RTD Out 0":cluster{"x":dbl, "y":dbl}[])  [unwired: 9 in]
            }
            frame #3 {
              n606 = call "Array_Search_For_Num.vi"("N Rows of Data"=w1115, "Title?"="Tc_down" ("String")) -> ("number"=w1113:dbl)  [unwired: 12 in, 1 out]
              "TcDown 0" <- w1113
            }
          }
          n607 = local read "RTDin to Downspout Offset"() -> (w1046:dbl)
          n608 = local read "Adj Time"() -> (w1044:dbl)
          n609 = local read "K(0.1)"() -> (w1045:dbl)
          n610 = local read "TempAdj"() -> (w1051:dbl)
          n611 = local read "MW100"() -> (w1053:refnum<visa-resource-name>)
          n612 = local read "Temperature Schedule"() -> (w1040:dbl[])
          n613 = local read "Flow Rate Schedule"() -> (w1039:dbl[])
          n614 = local read "DrawCount"() -> (w1038:i32)
          n615 = call "String_in_Reference.vi"("String"="Draw until heating turns on." ("string")) -> ()  [unwired: 18 in, 1 out]
          n616 = Index Array(array=w1039, index=w1038) -> (element=w1037:dbl)
          n617 = Index Array(array=w1040, index=w1038) -> (element=w1036:dbl)
          n618 = Subtract(x=w1036, y=w1046) -> (x-y=w1052:dbl)
          n619 = call "HEWH Temp Adjustment.vi"("VISA session"=w1053, "Semiphore"=w1065, "Degrees Target(58)"=w1052, "Degrees reading"=w1049, "Degrees setting In"=w1051, "Error In"=w1056, "Elapsed Time (sec)"=w1041, "Temp Adjust Time (3s)"=w1044, "K(0.1)"=w1045) -> ("VISA session out"=w1054:refnum<visa-resource-name>, "Degree setting Out"=w1050:dbl, "Error Out"=w1055:errorcluster)  [unwired: 4 in]
          n620 = local write "TempAdj"(w1050) -> ()
          n621 = call "HEWH Flow Adjustment.vi"("VISA session"=w1054, "Semiphore"=w1065, "GPM Target(3)"=w1037, "GPM reading"=w1048, "Flow rate setting In"=w1070, "Error In"=w1055, "Elapsed Time (sec)"=w1041, "Flow Adjust Time (3s)"=w1044, "K(0.1)"=w1045) -> ("Flow rate setting Out"=w1066:dbl, "Error Out"=w1063:errorcluster)  [unwired: 4 in, 1 out]
          n622 = local read "Stop Test Seqence"() -> (w1057:bool)
          n623 = disable-structure shown="Enabled" {
            disable-tunnel: [w1076 w1077 w1084 _] -> w1062
            disable-tunnel: [w1075 w1077 w1083 _] -> w1061
            disable-tunnel: [w1074 w1077 w1082 _] -> w1060
            disable-tunnel: [w1073 w1079 w1081 _] -> w1059
            disable-tunnel: w1042 -> [w1072 w1078 w1080 _]
            frame Disabled {
              n624 = Unbundle(w1072) -> ("UE"=w1073:bool, "LE"=w1074:bool, "COMP"=w1075:bool, "FANS"=w1076:bool)
            }
            frame Disabled {
              n625 = Unbundle(w1078) -> ("UE"=w1079:bool, "LE"=w1077:bool)  [unwired: 2 out]
            }
            frame Enabled {
              n626 = Unbundle(w1080) -> ("UE"=w1081:bool, "LE"=w1082:bool, "COMP"=w1083:bool, "FANS"=w1084:bool)
            }
            frame Disabled {
            }
          }
          n627 = Unbundle By Name(w1063) -> ("status"=w1069:bool)
          n628 = local write "Flow Adj"(w1066) -> ()
          n629 = local read "T5"() -> (w1067:u32)
          n630 = Compound Arithmetic op=OR(w1059, w1060, w1061, w1062, w1069, w1057, "Skip Draw0") -> (w1071:bool)
          n631 = Wait (ms)(milliseconds to wait=w1067) -> ()  [unwired: 1 out]
        }
      }
      frame "Term Draw" {
        # "For the Macro, we need Term Draw, and Draw Result in consecutive lines of data.  Thus the \"drawing\" semiphore flag."
        # "Energy(Wh)"
        n632 = flat-sequence {
          tunnel: [w1153] -> w1120
          tunnel: w1119 -> [w1153]
          frame #0 {
            n633 = local write "Drawing"(TRUE ("Drawing")) -> ()
          }
        }
        n634 = local read "Expansion Tank?"() -> (w1125:bool)
        n635 = local read "MW100"() -> (w1122:refnum<visa-resource-name>)
        n636 = call "HEWH Set Valves.vi"("VISA session"=w1122, "Semiphore"=w1123, "Expansion Tank?"=w1125, "Valve Bank Setting"=ValveBankPositions."Heating", "Error In"=w1120) -> ("Error Out"=w1124:errorcluster)  [unwired: 9 in, 1 out]
        n637 = local read "Calibration File Array"() -> (w1116:dbl[][])
        n638 = call "HEWH Totalize Flow Control.vi"("VISA session"=w1122, "Semiphore"=w1123, "Totalize Flow"=FALSE, "error in (no error)"=w1124) -> ("error out"=w1127:errorcluster)  [unwired: 10 in, 1 out]
        n639 = local read "Serial Data In"() -> (w1130:string)
        n640 = local read "Use Agilent?"() -> (w1131:bool)
        n641 = local read "Label Array"() -> (w1129:string[])
        n642 = local read "Equipment"() -> (w1134:T1)
        n643 = local read "Chanel List"() -> (w1142:string)
        n644 = local read "Semiphore"() -> (w1141:T2)
        n645 = control-ref of="Tank Display"() -> (w1143:refnum<vi>)
        n646 = call "Gather Test Data - Heatup Test new.vi"("Agilent Scan List"=w1142, "Semiphore"=w1141, "Equipment"=w1134, "Tank Display Ref"=w1143, "Agilent?"=w1131, "Calibration Coefficients"=w1116, "error in (no error)"=w1127, "Serial Data In"=w1130, "Agilent Label Array"=w1129) -> ("Output Data"=w1132:string[][], "POWER"=w1128:T4, "Voltage"=w1135:dbl, "error out"=w1133:errorcluster)  [unwired: 1 in, 2 out]
        n647 = local write "Voltage"(w1135) -> ()
        n648 = local read "Discard Last Draw"() -> (w1144:bool)
        n649 = local write "POWER"(w1128) -> ()
        n650 = Index Array(array=w1132, index (row)=1) -> (element=w1138:string[])  [unwired: 1 in]
        n651 = local read "FileName"() -> (w1136:path)
        n652 = call-poly <vilib>:"Write To Spreadsheet File.vi"("delimiter (\\t)"="," ("delimiter (\\t)"), "append to file? (new file:F)"=TRUE, "1D data"=w1138, "file path (dialog if empty)"=w1136) -> ()  [unwired: 4 in, 1 out]
        n653 = case shown="False" w1144 {
          tunnel: [w1171 w1176] -> w1146
          tunnel: w1145 -> [w1170 w1176]
          tunnel: [w1163 w1175] -> w1118
          tunnel: w1133 -> [w1154 w1175]
          tunnel: w1123 -> [_ _]
          tunnel: w1132 -> [w1157 _]
          frame False {
            n654 = local read "Volume(Gal.)"() -> (w1159:dbl)
            n655 = call "Array_Search_For_Num.vi"("N Rows of Data"=w1157, "Title?"="Energy(Wh)") -> ("number"=w1155:dbl)  [unwired: 12 in, 1 out]
            "WattHours" <- w1155
            n656 = local read "Total Gallons Drawn"() -> (w1160:dbl)
            n657 = local read "T*Max"() -> (w1172:dbl)
            n658 = local read "T*Ave"() -> (w1173:dbl)
            n659 = local read "T*min"() -> (w1174:dbl)
            n660 = call "E-Time.vi"("error in (no error)"=w1154) -> ("error out"=w1163:errorcluster, "Elapsed Time (sec)"=w1164:dbl)  [unwired: 8 in, 1 out]
            n661 = Add(x=w1159, y=w1160) -> (x+y=→"Total Gallons Drawn":dbl)
            n662 = Build Array(w1164, w1174, w1173, w1172, w1159, w1155) -> (w1169:dbl[])
            n663 = Build Array (concatenate)(w1170, w1169) -> (w1171:dbl[][])
            n664 = Number To Fractional String(number=w1169) -> (F-format string=w1167:string[])  [unwired: 3 in]
            n665 = local read "FileName"() -> (w1162:path)
            n666 = Build Array (concatenate)("Draw Result(time;T*min;T*ave;T*max; Volume(Gal. for M*);WattHours)", w1167) -> (w1166:string[])
            n667 = call-poly <vilib>:"Write To Spreadsheet File.vi"("delimiter (\\t)"="," ("delimiter (\\t)"), "append to file? (new file:F)"=TRUE, "1D data"=w1166, "file path (dialog if empty)"=w1162) -> ()  [unwired: 4 in, 1 out]
          }
          frame True {
          }
        }
        n668 = flat-sequence {
          tunnel: [w1151] -> w1117
          tunnel: w1118 -> [w1151]
          frame #0 {
            n669 = local write "Drawing"(FALSE ("Drawing")) -> ()
          }
        }
        n670 = case shown="Error" w1117 {
          selector: w1117 -> [w1177 w1180]
          tunnel: [w1178 string[] ["Finish"] ("States")] -> w1148
          tunnel: w1149 -> [w1178 _]
          tunnel: [w1177 w1180] -> w1147
          frame No Error {
          }
          frame Error {
          }
        }
      }
      frame "Finish", Default {
        n671 = local write "Status Tabl"(8 ("index")) -> ()
        n672 = case shown="No Error" w1184 {
          selector: w1184 -> [w1202 w1219]
          tunnel: [w1208 w1222] -> w1197
          tunnel: w1196 -> [w1208 w1222]
          tunnel: [w1203 errorcluster {"status"=FALSE, "code"=0, "source"=""} ("error IO")] -> w1186
          tunnel: w1182 -> [w1204 _]
          frame No Error {
            n673 = Equal?(x=w1204, y="Finish") -> (x = y?=w1207:bool)
            n674 = Concatenate Strings("False State: " ("string"), w1204) -> (w1201:string)
            n675 = case shown="True" w1207 {
              tunnel: [w1209 w1212] -> w1203
              tunnel: w1202 -> [w1209 w1211]
              tunnel: w1201 -> [_ w1210]
              frame True {
              }
              frame False {
                n676 = Bundle(cluster=w1211, "source"=w1210) -> (w1212:errorcluster)  [unwired: 2 in]
              }
            }
          }
          frame Error {
            n677 = Unbundle(w1219) -> ("code"=w1217:i32, "source"=w1214:string)  [unwired: 1 out]
            n678 = Number To Exponential String(number=w1217) -> (E-format string=w1216:string)  [unwired: 3 in]
            n679 = Concatenate Strings("ERROR: ", w1216, ": " ("string"), w1214) -> (w1213:string)
            n680 = local read "FileName"() -> (w1220:path)
            n681 = call "Log String to Spreadsheet.vi"("String"=w1213, "FileName"=w1220) -> ()  [unwired: 9 in, 1 out]
          }
        }
        n682 = Unbundle By Name(w1195) -> ("MW100"=w1187:refnum<visa-resource-name>)
        n683 = call "YKMW100 Get Error Log.vi"("VISA session"=w1187, "Semiphore"=w1181, "error in (no error)"=w1186) -> ("dup VISA session"=w1191:refnum<visa-resource-name>, "Error History"=→"Error History":string[], "error out"=w1192:errorcluster)  [unwired: 9 in, 1 out]
        n684 = call "YKMW100 Get Com Log.vi"("VISA session"=w1191, "Semiphore"=w1181, "error in (no error)"=w1192) -> ("Com History"=→"Com History":string[], "error out"=w1188:errorcluster)  [unwired: 9 in, 2 out]
        n685 = flat-sequence {
          tunnel: w1188 -> [w1199]
          tunnel: [w1199] -> w1185
          tunnel: w1185 -> [_]
          tunnel: w1184 -> [w1200]
          tunnel: [w1200] -> w1183
          frame #0 {
            w1198 = TRUE ("Stop Logging")
            n686 = local write "Stop Logging"(w1198) -> ()
            n687 = property on="Stop Logging" class="Bool (strict)"("Val(Sgnl)"=w1198) -> ()  [unwired: 2 in, 2 out]
          }
          frame #1 {
          }
        }
      }
    }
    n688 = Build Array (concatenate)(w43, w35) -> (w42:string[])
    "Executaion Sequence" <- w42
    n689 = Equal?(x=w35, y="Finish") -> (x = y?=w52:bool)
    n690 = local read "T2"() -> (w44:u32)
    n691 = Wait (ms)(milliseconds to wait=w44) -> ()  [unwired: 1 out]
  }
  "Error Out" <- w17
  "Test Data" <- w14
  n692 = event shown="[1] \"Init Complete\", \"Stop Logging\": Value Change" {
    selector: _ -> [_ _]
    dyn-events: _ -> [_ _]
    timeout: _ -> [_ _]
    event Timeout {
      n693 = event-data() -> ()  [unwired: 1 in, 2 out]
    }
    event "Init Complete", "Stop Logging": Value Change {
      n694 = local read "Serial Port Available?"() -> (w1223:bool)
      n695 = event-data() -> ()  [unwired: 1 in, 5 out]
      n696 = local read "COM Port"() -> (w1225:refnum<visa-resource-name>)
      n697 = while {
        tunnel: w1225 -> [w1233]
        tunnel: [w1231] -> w1224
        tunnel: w1223 -> [w1226]
        stop <- w1231 stop-if-true
        n698 = local read "Init Complete"() -> (w1228:bool)
        n699 = local read "GEA2 HyperData"() -> (w1227:bool)
        n700 = local read "PowerON"() -> (w1230:bool)
        n701 = And(x=w1226, y=w1228) -> (x .and. y?=w1229:bool)
        n702 = case shown="True" w1229 {
          selector: w1229 -> [_ w1239]
          tunnel: w1233 -> [_ w1243]
          tunnel: w1230 -> [_ w1240]
          tunnel: w1227 -> [_ w1235]
          frame False {
          }
          frame True {
            n703 = And(x=w1239, y=w1240) -> (x .and. y?=w1234:bool)
            n704 = Select(t=10, s=w1235, f=1) -> (s? t:f=w1236:i32)
            n705 = call "HEWH Serial Data Read.vi"("Serial Port Ref"=w1243, "GEA2 HyperData"=w1235, "Retries"=w1236, "Serial Port Available?"=w1234) -> ("Read String"=w1241:string, "error out"=→"Serial Error Out":errorcluster)  [unwired: 8 in, 2 out]
            n706 = local write "Serial Data In"(w1241) -> ()
          }
        }
        n707 = Wait (ms)(milliseconds to wait=u32 250) -> ()  [unwired: 1 out]
        n708 = local read "Stop Logging"() -> (w1231:bool)
      }
      "StopSerial" <- w1224
      n709 = property on="StopSerial" class="Bool (strict)"("Val(Sgnl)"=w1224) -> ()  [unwired: 2 in, 2 out]
    }
  }
  n710 = while {
    shift-right: [w1253] -> w12
    shift-left: 0 ("milliseconds to wait") -> [w1254]
    shift-right: [w1248] -> _
    shift-left: 0.0 -> [w1244]
    stop <- w1251 stop-if-true
    # "continuous data gathering"
    n711 = local read "Init Complete"() -> (w1255:bool)
    n712 = Multiply(x="Sample Per.(s)", y=1000.0) -> (x*y=w1245:dbl)
    n713 = local read "T2"() -> (w1256:u32)
    n714 = case shown="True" w1255 {
      tunnel: w1254 -> [w1264 w1276]
      tunnel: [w1264 w1275] -> w1253
      tunnel: [w1263 w1274] -> w1249
      tunnel: w1245 -> [_ w1271]
      tunnel: w1244 -> [_ w1268]
      frame False {
        (unwired) FALSE ("status")
        n715 = call "E-Time.vi"() -> ("Elapsed Time (sec)"=w1263:dbl)  [unwired: 9 in, 2 out]
      }
      frame True {
        n716 = To Long Integer(number=w1271) -> (32bit integer=w1266:i32)
        n717 = Multiply(x=w1268, y=1000.0) -> (x*y=w1270:dbl)
        n718 = To Long Integer(number=w1270) -> (32bit integer=w1267:i32)
        n719 = Subtract(x=w1266, y=w1267) -> (x-y=w1265:i32)
        n720 = In Range and Coerce(upper limit=w1266, x=w1265, lower limit=0) -> (coerced(x)=w1273:i32)  [unwired: 1 out]
        n721 = event shown="[0] Timeout" {
          selector: _ -> [_]
          dyn-events: _ -> [_]
          timeout: w1273 -> [_]
          tunnel: w1276 -> [w1283]
          tunnel: [w1280] -> w1275
          tunnel: [w1279] -> w1274
          event Timeout {
            # "Power Assumed to be on"
            n722 = event-data() -> ()  [unwired: 1 in, 2 out]
            n723 = local read "Calibration File Array"() -> (w1277:dbl[][])
            n724 = flat-sequence {
              tunnel: [w1323] -> w1282
              tunnel: [w1322] -> w1281
              tunnel: [w1321] -> w1279
              frame #0 {
                n725 = local read "Serial Data In"() -> (w1323:string)
                n726 = local read "Label Array"() -> (w1322:string[])
                n727 = call "E-Time.vi"() -> ("Elapsed Time (sec)"=w1321:dbl)  [unwired: 9 in, 2 out]
              }
            }
            n728 = local read "Use Agilent?"() -> (w1311:bool)
            n729 = local read "Semiphore"() -> (w1313:T2)
            n730 = local read "Equipment"() -> (w1314:T1)
            n731 = local read "Chanel List"() -> (w1312:string)
            n732 = control-ref of="Tank Display"() -> (w1310:refnum<vi>)
            n733 = call "Gather Test Data - Heatup Test new.vi"("Agilent Scan List"=w1312, "Semiphore"=w1313, "Equipment"=w1314, "Tank Display Ref"=w1310, "Agilent?"=w1311, "Calibration Coefficients"=w1277, "Serial Data In"=w1282, "Agilent Label Array"=w1281) -> ("Tc Tree"=w1301:dbl[], "Output Data"=w1284:string[][], "POWER"=w1278:T4, "PowerData"=w1300:T24, "Voltage"=→"Voltage":dbl, "error out"=→"Error Datalogging":errorcluster)  [unwired: 2 in]
            "Log Data" <- w1284
            n734 = local write "POWER"(w1278) -> ()
            n735 = Array To Cluster(array=w1301) -> (cluster=w1291:T22)
            n736 = Unbundle(w1278) -> ("UE"=w1298:bool, "LE"=w1296:bool, "COMP"=w1297:bool, "FANS"=w1308:bool)
            n737 = Build Array(w1291) -> (→"Temps":T8)
            n738 = Boolean To (0,1)(Boolean=w1308) -> (0, 1=w1309:i16)
            n739 = Boolean To (0,1)(Boolean=w1298) -> (0, 1=w1303:i16)
            n740 = Boolean To (0,1)(Boolean=w1297) -> (0, 1=w1307:i16)
            n741 = Boolean To (0,1)(Boolean=w1296) -> (0, 1=w1305:i16)
            n742 = Unbundle By Name(w1300) -> ("Power"=w1302:dbl)
            n743 = Increment(x=w1283) -> (x+1=w1280:i32)
            "Number of Records" <- w1280
            n744 = expression code="2*x"(w1307) -> (w1289:i16)
            n745 = Index Array(array=w1284, index (row)=1) -> (element=w1285:string[])  [unwired: 1 in]
            n746 = expression code="3*x"(w1305) -> (w1306:i16)
            n747 = expression code="4*x"(w1303) -> (w1304:i16)
            n748 = call "Array_Search_For_Num.vi"("N Rows of Data"=w1284, "Title?"="GALLONS") -> ("number"=→"Gallons Chart":dbl)  [unwired: 12 in, 1 out]
            n749 = Build Array(w1302, w1304, w1306, w1289, w1309) -> (w1293:dbl[])
            n750 = Array To Cluster(array=w1293) -> (cluster=w1295:T26)
            n751 = flat-sequence {
              tunnel: w1285 -> [w1316]
              frame #0 {
                # "Dont record during draw"
                n752 = local read "Drawing"() -> (w1315:bool)
                n753 = case shown="False" w1315 {
                  tunnel: w1316 -> [w1319 _]
                  frame False {
                    n754 = local read "FileName"() -> (w1320:path)
                    n755 = call-poly <vilib>:"Write To Spreadsheet File.vi"("delimiter (\\t)"="," ("delimiter (\\t)"), "append to file? (new file:F)"=TRUE, "1D data"=w1319, "file path (dialog if empty)"=w1320) -> ()  [unwired: 4 in, 1 out]
                  }
                  frame True {
                  }
                }
              }
            }
            n756 = Build Array(w1295) -> (→"Watt Chart":T10)
          }
        }
      }
    }
    n757 = Wait (ms)(milliseconds to wait=w1256) -> ()  [unwired: 1 out]
    n758 = disable-structure shown="Enabled" {
      disable-tunnel: [w1257 FALSE ("status")] -> w1250
      frame Disabled {
        n759 = local read "Error Datalogging"() -> (w1258:errorcluster)
        n760 = Unbundle By Name(w1258) -> ("status"=w1257:bool)
      }
      frame Enabled {
      }
    }
    n761 = Or(x=w1250, y="Stop Logging") -> (x .or. y?=w1251:bool)
    n762 = flat-sequence {
      tunnel: w1249 -> [w1261]
      tunnel: [w1260] -> w1248
      frame #0 {
        n763 = call "E-Time.vi"() -> ("Elapsed Time (sec)"=w1262:dbl)  [unwired: 9 in, 2 out]
        n764 = Subtract(x=w1262, y=w1261) -> (x-y=w1260:dbl)
      }
    }
  }
  n765 = while {
    stop <- w1325 stop-if-true
    n766 = local read "T3"() -> (w1326:u32)
    n767 = To Long Integer(number=w1326) -> (32bit integer=w1324:i32)
    n768 = event shown="[1] \"stop\": Value Change" {
      selector: _ -> [_ _ _ _ _]
      dyn-events: _ -> [_ _ _ _ _]
      timeout: w1324 -> [_ _ _ _ _]
      tunnel: [_ "stop" _ _ _] -> w1325
      event Timeout {
        n769 = event-data() -> ()  [unwired: 1 in, 2 out]
        n770 = stacked-sequence {
          frame #0 {
            n771 = call "String_in_Reference.vi"() -> ("String Out"=→"STATUS":string)  [unwired: 19 in]
            n772 = call "E-Time.vi"() -> ("Elapsed Time (sec)"=→"Elapsed.Time (H:M:S)":dbl)  [unwired: 9 in, 2 out]
          }
          frame #1 {
            n773 = local read "Log Data"() -> (w1345:string[][])
            n774 = Index Array(array=w1345, index (row)=1) -> (element=w1346:string[])  [unwired: 1 in]
            n775 = Fract/Exp String To Number(string=w1346) -> (number=w1330:dbl[])  [unwired: 3 in, 1 out]
            n776 = Index Array(array=w1330, index #1="P1", index #2="P5", index #3="T1 2", index #4="T2 2", index #5="T5 2", index #6=0 ("index"), index #7="P2") -> (element #1=w1343:dbl, element #2=w1340:dbl, element #3=w1339:dbl, element #4=w1338:dbl, element #5=w1337:dbl, element #6=→"Time":dbl, element #7=w1329:dbl)
            n777 = call "R134a-PH Curves.vi"("P1 (Compressor In, P Low)"=w1343, "P2 (Compressor Out, P High1)"=w1329, "P5 (Expansion In, P High2)"=w1340, "T1 (Compressor In, T3B)"=w1339, "T2 Compressor Out, T4)"=w1338, "T6 (Evap In, T3A)"=w1337) -> ("XY Graph"=→"XY Graph":cluster{dbl[], dbl[]}[], "P-T-H Data"=→"P-T-H Data 2":dbl[][])  [unwired: 8 in]
          }
        }
      }
      event "stop": Value Change {
        n778 = event-data() -> ()  [unwired: 1 in, 5 out]
        n779 = case shown="True" "stop" {
          frame False {
          }
          frame True {
            n780 = stacked-sequence {
              frame #0 {
                w1357 = T25 30 items=["4-20_OUT", "Pres_HI1", "Pres_HI2", "Pres_LOW", "Pres_PIN", "HEATER_TOP", "HEATER_BOT", "T_Shell", "FLOWMETER", "WATT_SENSE", "WH_TICK", "Tc_1", "Tc_2", "Tc_3", "Tc_4", "Tc_5", "Tc_6", "Tc_down", "T_Shell_2", "T_Shell_3", "T_Shell_4", "RTD_IN", "RTD_OUT", "RTD_AMB", "INTF_TEMPFLO", "INTF_READY", "INTF_START", "INTF_STOP", "DRM_LOW", "DRM_HIGH", "PWR_MAIN", "VLV_DUMP", "VLV_OUT", "VLV_IN", "WATT_HOURS", "FLOW(SAMPLE)", "GALLONS", "FLOW(GPM)"] ("Channel_Enum")
                # "Turn off water, and power on, open output valve"
                n781 = local read "Expansion Tank?"() -> (w1353:bool)
                n782 = local read "Semiphore"() -> (w1354:T2)
                n783 = local read "MW100"() -> (w1351:refnum<visa-resource-name>)
                n784 = call "HEWH Set Valves.vi"("VISA session"=w1351, "Semiphore"=w1354, "Expansion Tank?"=w1353, "Valve Bank Setting"=ValveBankPositions."Resting") -> ("dup VISA session"=w1355:refnum<visa-resource-name>, "Error Out"=w1356:errorcluster)  [unwired: 10 in]
                n785 = local write "STATUS"("Stopping Test..." ("string")) -> ()
                n786 = call "Generic - DO1.vi"("VISA session"=w1355, "Semiphore"=w1354, "Channel_Enum"=w1357, "Relay Status (0:CLOSED)"=enum8{"CLOSED", "OPEN"}."OPEN", "Error In"=w1356) -> ()  [unwired: 9 in, 2 out]
              }
              frame #1 {
                n787 = local read "Error Datalogging"() -> (w1360:errorcluster)
                n788 = Unbundle By Name(w1360) -> ("status"=w1359:bool)
                n789 = case shown="True" w1359 {
                  frame False {
                  }
                  frame True {
                    n790 = local read "FileName"() -> (w1361:path)
                    n791 = call "Log String to Spreadsheet.vi"("String"="Error Datalogging", "FileName"=w1361) -> ()  [unwired: 9 in, 1 out]
                  }
                }
              }
              frame #2 {
                n792 = local read "Serial Data In"() -> (w1366:string)
                n793 = local read "Use Agilent?"() -> (w1367:bool)
                n794 = local read "Equipment"() -> (w1376:T1)
                n795 = local read "Chanel List"() -> (w1378:string)
                n796 = local read "Label Array"() -> (w1365:string[])
                n797 = local read "Semiphore"() -> (w1377:T2)
                n798 = control-ref of="Tank Display"() -> (w1379:refnum<vi>)
                n799 = local read "FileName"() -> (w1369:path)
                n800 = local read "Calibration File Array"() -> (w1363:dbl[][])
                n801 = call "Gather Test Data - Heatup Test new.vi"("Agilent Scan List"=w1378, "Semiphore"=w1377, "Equipment"=w1376, "Tank Display Ref"=w1379, "Agilent?"=w1367, "Calibration Coefficients"=w1363, "Serial Data In"=w1366, "Agilent Label Array"=w1365) -> ("Output Data"=w1375:string[][], "POWER"=w1364:T4, "Voltage"=w1380:dbl)  [unwired: 2 in, 3 out]
                n802 = local write "POWER"(w1364) -> ()
                n803 = Index Array(array=w1375, index (row)=1) -> (element=w1372:string[])  [unwired: 1 in]
                n804 = call-poly <vilib>:"Write To Spreadsheet File.vi"("delimiter (\\t)"="," ("delimiter (\\t)"), "append to file? (new file:F)"=TRUE, "1D data"=w1372, "file path (dialog if empty)"=w1369) -> ("new file path (Not A Path if cancelled)"=w1368:path)  [unwired: 4 in]
                n805 = local write "Voltage"(w1380) -> ()
                n806 = call "Log String to Spreadsheet.vi"("String"="Stopped", "FileName"=w1368) -> ()  [unwired: 9 in, 1 out]
              }
              frame #3 {
                n807 = local read "Init Complete"() -> (w1382:bool)
                n808 = local read "Local?"() -> (w1381:bool)
                n809 = And(x=w1381, y=w1382) -> (x .and. y?=w1383:bool)
                n810 = case shown="True" w1383 {
                  tunnel: w1381 -> [_ w1384]
                  frame False {
                  }
                  frame True {
                    n811 = local read "Equipment"() -> (w1387:T1)
                    n812 = local read "Semiphore"() -> (w1386:T2)
                    n813 = call "HEWH CloseEquipmet.vi"("Semiphore"=w1386, "Equipment"=w1387) -> ("Error Out"=w1385:errorcluster)  [unwired: 9 in]
                    n814 = call "Semiphore-Destroy-Local.vi"("Semiphore"=w1386, "Local?"=w1384, "error in (no error)"=w1385) -> ()  [unwired: 16 in, 1 out]
                  }
                }
              }
              frame #4 {
                n815 = local read "FileName"() -> (w1389:path)
                n816 = call <vilib>:"Check if File or Folder Exists.vi"("path"=w1389) -> ("file or folder exists?"=w1388:bool)  [unwired: 8 in, 2 out]
                n817 = case shown="True" w1388 {
                  tunnel: w1389 -> [_ w1394]
                  frame False {
                  }
                  frame True {
                    n818 = Strip Path(path=w1394) -> (name=w1393:string)  [unwired: 1 out]
                    n819 = Search and Replace String(input string=w1393, search string=".tmp", replace string=".csv" ("search string")) -> (result string=w1391:string, error out=w1397:errorcluster)  [unwired: 5 in, 2 out]
                    n820 = Build Path(base path="Save File Directory", name or relative path=w1391) -> (appended path=w1390:path)
                    n821 = local write "FileName"(w1390) -> ()
                    n822 = Move(source path=w1394, error in=w1397, 10:w1390) -> ()  [unwired: 2 in, 3 out]
                  }
                }
              }
              frame #5 {
                n823 = local read "Computer Name"() -> (w1398:string)
                n824 = local read "Ver."() -> (w1399:string)
                n825 = property class="App"() -> ("App.Name"=w1402:string)  [unwired: 2 in, 2 out]
                n826 = local read "LAN IP Address"() -> (w1403:string)
                n827 = call <vilib>:"Space Constant.vi"() -> ("String"=w1401:string)
                n828 = Concatenate Strings(w1403, w1401, w1398, w1401, w1402, w1401, w1399, w1401, "Completed." ("string")) -> (w1404:string)
                n829 = call "Save Time to File.vi"("String"=w1404) -> ()  [unwired: 13 in, 2 out]
              }
              frame #6 {
                n830 = global read "Global HEWH.vi" "Test Station:"() -> (w1406:string)
                n831 = Concatenate Strings("robocopy c:/Data //10.2.0.10/AP2Lab/" ("command line"), w1406) -> (w1405:string)
                n832 = call <vilib>:"System Exec.vi"("command line"=w1405) -> ()  [unwired: 7 in, 4 out]
              }
              frame #7 {
                n833 = event shown="[1] \"StopSerial\": Value Change" {
                  selector: _ -> [_ _]
                  dyn-events: _ -> [_ _]
                  timeout: _ -> [_ _]
                  event Timeout {
                    n834 = event-data() -> ()  [unwired: 1 in, 2 out]
                  }
                  event "StopSerial": Value Change {
                    w1408 = FALSE ("stop")
                    n835 = event-data() -> ()  [unwired: 1 in, 5 out]
                    n836 = local write "Stop Logging"(w1408) -> ()
                    n837 = property on="Stop Logging" class="Bool (strict)"("Val(Sgnl)"=w1408) -> ()  [unwired: 2 in, 2 out]
                    n838 = local write "STATUS"("Stopped OK" ("STATUS")) -> ()
                  }
                }
              }
            }
          }
        }
      }
      event "Help": Value Change {
        n839 = event-data() -> ()  [unwired: 1 in, 5 out]
        n840 = One Button Dialog(message="\n10 CFR part 430 5.1.4 First-Hour Rating Test\n5.1.4.3.P1.2\tWater heater not operating, initiate a draw\n5.1.4.3.P1.3\tTerminate draw after cut in of the upper most element\n5.1.4.3.P1.4\tAfter cut out, monitor 6 internal Tcs every minute\n5.1.4.3.P2.1\tInitiate draw After cut out and average tank temp is max\n5.1.4.3.P2.2\tRecord output water temp after 15 secs, and at 5 sec intervals thereafter\n5.1.4.3.P2.3\tMonitor inlet water temp, must be 58 +/- 2 F\n5.1.4.3.P2.4\tTerminate draw when ouytput temp = T*max -25F, record T*min\n5.1.4.3.P2.5\tRecord ave output water temp, Mass/volumt removed\n5.1.4.3.P3.1\tPerform second draw when eletricity to heating is reduced\n5.1.4.3.P4\tRepeat for 1 hour\n\tLast draw: there are special cases\n5.1.4.3.P5.1\tA  draw is going at t-1 hr, complete\n5.1.4.3.P5.1.5\tIf a draw is not going, immediately start and continue for at least 30 seconds\n5.1.4.3.P5.1.6\t If after 30 sec, T< last tmin, stop and discard measurements, else continue\n") -> (true=w1411:bool)  [unwired: 1 in]
        n841 = Not(x=w1411) -> (.not. x?=w1410:bool)
        n842 = local write "Help"(w1410) -> ()
      }
      event "Time Reset": Value Change {
        n843 = event-data() -> ()  [unwired: 1 in, 5 out]
        n844 = call "E-Time.vi"("Set Start Time (s)"="Time Update", "Reset"="Time Reset") -> ("error out"=w1413:errorcluster)  [unwired: 7 in, 2 out]
        n845 = flat-sequence {
          tunnel: w1413 -> [_]
          frame #0 {
            n846 = local write "Time Reset"(FALSE ("Time Reset")) -> ()
          }
        }
      }
      event Value Change {
        n847 = event-data() -> ()  [unwired: 1 in, 5 out]
        n848 = local read "Serial Data In"() -> (w1428:string)
        n849 = local read "Use Agilent?"() -> (w1429:bool)
        n850 = local read "Label Array"() -> (w1427:string[])
        n851 = local read "Equipment"() -> (w1431:T1)
        n852 = local read "Chanel List"() -> (w1433:string)
        n853 = local read "Semiphore"() -> (w1432:T2)
        n854 = control-ref of="Tank Display"() -> (w1434:refnum<vi>)
        n855 = local read "FileName"() -> (w1420:path)
        n856 = local read "Calibration File Array"() -> (w1417:dbl[][])
        n857 = call "Gather Test Data - Heatup Test new.vi"("Agilent Scan List"=w1433, "Semiphore"=w1432, "Equipment"=w1431, "Tank Display Ref"=w1434, "Agilent?"=w1429, "Calibration Coefficients"=w1417, "Serial Data In"=w1428, "Agilent Label Array"=w1427) -> ("Output Data"=w1426:string[][], "POWER"=→"POWER":T4, "Voltage"=w1430:dbl)  [unwired: 2 in, 3 out]
        n858 = local write "Voltage"(w1430) -> ()
        n859 = local write "Log Data"(w1426) -> ()
        n860 = Index Array(array=w1426, index (row)=1) -> (element=w1423:string[])  [unwired: 1 in]
        n861 = call-poly <vilib>:"Write To Spreadsheet File.vi"("delimiter (\\t)"="," ("delimiter (\\t)"), "append to file? (new file:F)"=TRUE, "1D data"=w1423, "file path (dialog if empty)"=w1420) -> ("new file path (Not A Path if cancelled)"=w1419:path)  [unwired: 4 in]
        n862 = call "Log String to Spreadsheet.vi"("String"="Power Change", "FileName"=w1419) -> ()  [unwired: 9 in, 1 out]
      }
    }
  }
  n863 = flat-sequence {
    tunnel: w12 -> [_]
    frame #0 {
      w1435 = TRUE ("stop")
      n864 = property on="stop" class="Bool (strict)"("Val(Sgnl)"=w1435) -> ()  [unwired: 2 in, 2 out]
      n865 = local write "stop"(w1435) -> ()
    }
  }
